vi "SIAM-SIMStack_v3camphase.vi"(7 "Constants":T2={"galvox-Line0"=14800, "GalvoX-Blanking"=15000.0, "galvox-count/pix"=-2.47, "Camera-StartLine"=1, "Camera-Endline"=5000, "Wobbel-total"=4900.0, "SM_ticks"=116, "Trigger_ticks"=100, "galvoxAccel"=10.0, "WobbelAccel"=0.04, "zAccel"=0.05, "z-delay-ticks"=700, "SCMOS-LineSpeed [10µs]"=2.472, "RollingShutter height- Pix"=200} {"SCMOS-LineSpeed [10µs]" format="%#.6f" items=["Fast-285MHz"=0.9175, "Slow-95MHz"=2.7525, "Slow4.2"=2.7766]; "galvox-count/pix" format="%#_5f"}, 8 "error in (no error)":errorcluster, 11 "User":T3={"z-distance_nm"=-200, "#planes"=1, "Digital-out"=enum."Laser1", "NoOfPhaseImages"=7} {"#planes" min=1}) -> (0 "error out":errorcluster, 1 "SIAMScript":T5(array[cluster])=[{"Delay 10µs"=50, "command"=4060086273, "P0"=3, "P1"=1, "P2"=0, "P3"=0, "P4"=0, "P5-ticket"=0}, {"Delay 10µs"=0, "command"=101711937, "P0"=0, "P1"=160563200, "P2"=0, "P3"=0, "P4"=0, "P5-ticket"=0}, {"Delay 10µs"=0, "command"=102760513, "P0"=0, "P1"=985958318, "P2"=0, "P3"=0, "P4"=0, "P5-ticket"=0}, {"Delay 10µs"=0, "command"=3289190402, "P0"=0, "P1"=0, "P2"=0, "P3"=0, "P4"=0, "P5-ticket"=0}, {"Delay 10µs"=1, "command"=4076863488, "P0"=0, "P1"=381040, "P2"=0, "P3"=0, "P4"=0, "P5-ticket"=0}, {"Delay 10µs"=0, "command"=4076863492, "P0"=0, "P1"=0, "P2"=0, "P3"=0, "P4"=0, "P5-ticket"=0}, {"Delay 10µs"=0, "command"=4076863497, "P0"=0, "P1"=1, "P2"=0, "P3"=0, "P4"=0, "P5-ticket"=0}, {"Delay 10µs"=0, "command"=4076863494, "P0"=0, "P1"=0, "P2"=0, "P3"=0, "P4"=0, "P5-ticket"=0}, {"Delay 10µs"=0, "command"=4076863488, "P0"=0, "P1"=40, "P2"=0, "P3"=0, "P4"=0, "P5-ticket"=0}, {"Delay 10µs"=0, "command"=4060086273, "P0"=10, "P1"=-65, "P2"=0, "P3"=0, "P4"=0, "P5-ticket"=0}, {"Delay 10µs"=0, "command"=4076863492, "P0"=10, "P1"=0, "P2"=0, "P3"=0, "P4"=0, "P5-ticket"=0}, {"Delay 10µs"=264, "command"=102760481, "P0"=0, "P1"=0, "P2"=-1047728, "P3"=0, "P4"=0, "P5-ticket"=0}, {"Delay 10µs"=0, "command"=4060086273, "P0"=2, "P1"=7, "P2"=0, "P3"=0, "P4"=0, "P5-ticket"=0}, {"Delay 10µs"=116, "command"=3489660929, "P0"=2097152, "P1"=2097152, "P2"=0, "P3"=0, "P4"=0, "P5-ticket"=0}, {"Delay 10µs"=0, "command"=3489660929, "P0"=1, "P1"=1, "P2"=0, "P3"=0, "P4"=0, "P5-ticket"=0}, {"Delay 10µs"=100, "command"=3489660929, "P0"=1, "P1"=0, "P2"=0, "P3"=0, "P4"=0, "P5-ticket"=0}, {"Delay 10µs"=12638, "command"=3289190402, "P0"=0, "P1"=0, "P2"=0, "P3"=0, "P4"=0, "P5-ticket"=0}, {"Delay 10µs"=1, "command"=4076863488, "P0"=0, "P1"=381040, "P2"=0, "P3"=0, "P4"=0, "P5-ticket"=0}, {"Delay 10µs"=0, "command"=4076863492, "P0"=0, "P1"=0, "P2"=0, "P3"=0, "P4"=0, "P5-ticket"=0}, {"Delay 10µs"=0, "command"=4076863497, "P0"=0, "P1"=1, "P2"=0, "P3"=0, "P4"=0, "P5-ticket"=0}, {"Delay 10µs"=0, "command"=4076863494, "P0"=0, "P1"=0, "P2"=0, "P3"=0, "P4"=0, "P5-ticket"=0}, {"Delay 10µs"=0, "command"=4076863488, "P0"=0, "P1"=40, "P2"=0, "P3"=0, "P4"=0, "P5-ticket"=0}, {"Delay 10µs"=0, "command"=4060086273, "P0"=10, "P1"=-65, "P2"=0, "P3"=0, "P4"=0, "P5-ticket"=0}, {"Delay 10µs"=0, "command"=4076863492, "P0"=10, "P1"=0, "P2"=0, "P3"=0, "P4"=0, "P5-ticket"=0}, {"Delay 10µs"=0, "command"=102760465, "P0"=0, "P1"=794884, "P2"=0, "P3"=0, "P4"=0, "P5-ticket"=0}, {"Delay 10µs"=0, "command"=101711889, "P0"=0, "P1"=42448, "P2"=0, "P3"=0, "P4"=0, "P5-ticket"=0}, {"Delay 10µs"=132, "command"=102760465, "P0"=0, "P1"=-794884, "P2"=0, "P3"=0, "P4"=0, "P5-ticket"=0}, {"Delay 10µs"=0, "command"=101711889, "P0"=0, "P1"=-42448, "P2"=0, "P3"=0, "P4"=0, "P5-ticket"=0}, {"Delay 10µs"=132, "command"=102760465, "P0"=0, "P1"=0, "P2"=0, "P3"=0, "P4"=0, "P5-ticket"=0}, {"Delay 10µs"=0, "command"=101711889, "P0"=0, "P1"=0, "P2"=0, "P3"=0, "P4"=0, "P5-ticket"=0}, {"Delay 10µs"=12855, "command"=3489660929, "P0"=2097152, "P1"=0, "P2"=0, "P3"=0, "P4"=0, "P5-ticket"=0}, {"Delay 10µs"=70, "command"=4043379297, "P0"=-6, "P1"=2, "P2"=1, "P3"=0, "P4"=0, "P5-ticket"=514}, {"Delay 10µs"=50, "command"=104857729, "P0"=-25600, "P1"=0, "P2"=0, "P3"=0, "P4"=0, "P5-ticket"=0}, {"Delay 10µs"=0, "command"=4043379297, "P0"=-43, "P1"=3, "P2"=1, "P3"=0, "P4"=0, "P5-ticket"=515}, {"Delay 10µs"=50, "command"=104857729, "P0"=25600, "P1"=0, "P2"=0, "P3"=0, "P4"=0, "P5-ticket"=0}, {"Delay 10µs"=50, "command"=102760513, "P0"=0, "P1"=983040000, "P2"=0, "P3"=0, "P4"=0, "P5-ticket"=0}, {"Delay 10µs"=10, "command"=4027518991, "P0"=0, "P1"=0, "P2"=0, "P3"=0, "P4"=0, "P5-ticket"=112}] {"command" format="%x" items=["read_x-Motor_status_ticket"=17305600, "init_x-Motor"=17760263, "read_x-Motor_absolute_ticket"=16781312, "move_x-Motor_absolute"=16777217, "move_x-Motor_relative"=16842753, "read_x-Motor_speed"=16977920, "set_x-Motor_speed"=16973825, "read_y-Motor_status_ticket"=18354176, "init_y-Motor"=18808839, "read_y-Motor_absolute_ticket"=17829888, "move_y-Motor_absolute"=17825793, "move_y-Motor_relative"=17891329, "read_y-Motor_speed"=18026496, "set_y-Motor_speed"=18022401, "read_z-Motor_status_ticket"=19402752, "init_z-Motor"=19857415, "stop_z-Motor"=19857423, "start_z-Motor"=19857422, "read_z-Motor_absolute_ticket"=18878464, "move_z-Motor_absolute"=18874369, "move_z-Motor_relative"=18939905, "read_Objective_status_ticket"=20451328, "init_Objective"=20905991, "read_Objective_absolute_ticket"=19927040, "move_Objective_absolute"=19922945, "move_Objective_relative"=19988481, "read_Objective-Motor_speed"=20123648, "set_Objective-Motor_speed"=20119553, "read_Filter_status_ticket"=21499904, "init_Filter"=21954567, "read_Filter_absolute_ticket"=20975616, "move_Filter_absolute"=20971521, "move_Filter_relative"=21037057, "read_Filter-Motor_speed"=21172224, "set_Filter-Motor_speed"=21168129, "read_Trans-Rad_status_ticket"=22548480, "init_Trans-Rad"=23003143, "read_Trans-Rad_absolute_ticket"=22024192, "move_Trans-Rad_absolute"=22020097, "move_Trans-Rad_relative"=22085633, "read_Trans-Motor_speed"=22220800, "set_Trans-Motor_speed"=22216705, "read_FRET_status_ticket"=23597056, "init_FRET"=24051719, "read_FRET_absolute_ticket"=23072768, "move_FRET_absolute"=23068673, "move_FRET_relative"=23134209, "read_FRET-Motor_speed"=23269376, "set_FRET-Motor_speed"=23265281, "read_SI-Rad_status_ticket"=24645632, "init_SI-Rad"=25100295, "read_SI-Rad_absolute_ticket"=24121344, "move_SI-Rad_absolute"=24117249, "move_SI-Rad_relative"=24182785, "read_SI-Rad_speed"=24317952, "set_SI-Rad_speed"=24313857, "I2C-write"=335544337, "I2C-read"=335548433, "UART0-VC-Baud-write"=469958673, "UART0-VC-Baud-read"=469962768, "UART0-VC-write"=469762065, "UART0-VC-write-Var"=469762067, "UART0-VC-read"=469766160, "UART0-VC-read-Var"=469766162, "UART1-TSM-Baud-read"=486739984, "UART1-TSM-write"=486539281, "UART1-TSM-write-ticket"=486543377, "UART1-TSM-write-var-binary"=486539283, "UART1-TSM-write-var-binary-ticket"=486543379, "UART1-TSM-read"=486543376, "UART1-TSM-read-var-binary"=486543378, "UART2-write"=503316497, "UART2-read"=503320592, "USB-UART0-write"=536870929, "USB-UART0-read"=536875024, "USB-UART0-Float-Bitschift"=537133073, "USB-UART0-read-Float"=536875234, "USB-UART0-write-Float"=536871139, "USB-UART0-read-Float"=536875250, "USB-UART0-write-Float"=536871155, "end_no_ticket"=4027514895, "end_ticket"=4027518991, "IO-read_bank0"=3489665024, "IO-write_bank0"=3489660929, "IO-read_bank1"=3506442240, "IO-write_bank1"=3506438145, "DA0-0_LED365"=2684354561, "DA0-1_LED385"=2685403137, "DA0-2_LED440"=2686451713, "DA0-3_LED470"=2687500289, "DA0-4_LED510"=2688548865, "DA0-5_LED550"=2689597441, "DA0-6_LED590"=2690646017, "DA0-7_LED640"=2691694593, "DA1-0_LED-R"=2701131777, "DA1-1_LED-G"=2702180353, "DA1-2_LED-B"=2703228929, "DA1-3_LED-AF"=2704277505, "DA1-4"=2705326081, "DA1-5"=2706374657, "DA1-6"=2707423233, "DA1-7"=2708471809, "DA2-Laser0"=2717908993, "DA2-Laser1"=2718957569, "DA2-Laser2"=2720006145, "DA2-Laser3"=2721054721, "DA2-Laser4"=2722103297, "Analog-read_AD0-0"=2818576384, "Analog-read-store_AD0-0"=2818572290, "IO-delay_bank0"=3489923073, "IO-delay_bank0_fromVar"=3489923075, "read_cam_clock"=3289124864, "store_cam_clock"=3289120770, "read_cam_phase"=3289190400, "store_cam_phase"=3289186306, "store_cam_phase-t"=3289190402, "Read ticks"=4027518976, "Read ticks to var"=4027518978, "Read IP"=4043313152, "Read IP into var"=4043313154, "Set IP from var"=4043309059, "Set IP from var, relative"=4043313155, "decrement_branchRel_if_equal"=4043374945, "decrement_branchRel_if_greaterequal"=4043375201, "decrement_branchRel_if_greaterequal_withTicket"=4043379297, "decrement_branchRel_if_smaller"=4043375457, "increment_branchRel_if_smaller"=4043375473, "readVar"=4060090368, "writeVar"=4060086273, "copyVar0_from_var1"=4060086275, "math_addToVariable"=4076863488, "math_addVToVariable"=4076863489, "math_subToVariable"=4076863490, "math_subVToVariable"=4076863491, "math_multToVariable"=4076863492, "math_multvToVariable"=4076863493, "math_divideToVariable"=4076863494, "math_divideVToVariable"=4076863495, "math_modToVariable"=4076863496, "math_modVToVariable"=4076863497, "logic_and"=4093640704, "logic_or"=4093640706, "logic_xor"=4093640708, "bitshift"=4093640712, "set_1Galvo"=101712113, "set_x-Galvo"=102760689, "set_y-Galvo"=103809265, "set_z-Fokus"=104857841, "set_1Galvo_position-only"=101711937, "set_x-Galvo_position-only"=102760513, "set_y-Galvo_position-only"=103809089, "set_z-Fokus_position-only"=104857665, "set_x-Galvo_position-only_ticket"=102764609, "set_y-Galvo_position-only_ticket"=103813185, "set_z-Fokus_position-only_ticket"=104861761, "set_1Galvo_relativ-only"=101712001, "set_x-Galvo_relativ-only"=102760577, "set_y-Galvo_relativ-only"=103809153, "set_z-Fokus_relativ-only"=104857729, "set_1Galvo_speed-only"=101711905, "set_x-Galvo_speed-only"=102760481, "set_y-Galvo_speed-only"=103809057, "set_z-Fokus_speed-only"=104857633, "set_1Galvo_acc-only"=101711889, "set_x-Galvo_acc-only"=102760465, "set_y-Galvo_acc-only"=103809041, "set_z-Fokus_acc-only"=104857617, "read_1Galvo_ticket"=101716032, "read_x-Galvo_ticket"=102764608, "read_y-Galvo_ticket"=103813184, "read_z-Focus_ticket"=104861760, "x-Galvo_pos_fromVar"=102760515, "y-Galvo_pos_fromVar"=103809091, "z-Focus_pos_fromVar"=104857667, "Servo0"=67108865, "Servo0-enable"=68091911, "Servo0-disable"=68091919, "Servo1"=68157441, "Servo1-enable"=69140487, "Servo1-disable"=69140495, "Servo2-enable"=70189063, "Servo2"=69206017, "Servo3-enable"=71237639, "Servo3"=70254593, "xEncoder-Enable"=202309639, "xEncoder-Bits"=201523201, "xEncoder-Read"=201330688, "xEncoder-Read"=201326594, "xEncoder-Read-ticket"=201330690, "yEncoder-Enable"=203358215, "yEncoder-Bits"=202571777, "yEncoder-Read"=202379264, "yEncoder-Read"=202375170, "yEncoder-Read-ticket"=202379266]}, 2 "Camera":T1={"Camera-Exposure"=0.0, "CameraImages"=7})   [LabVIEW 2011]
uses:
  SIAM_command.ctl
panel:
  out "phase a":dbl=0.04048114735137636
  out "galvo a":dbl=0.7580607172293603
  out "GalvoMove":dbl=-12844.599514563108
  out "PredictionTime":u32=381
  out "FrameClock":u32=13119
  out "CamTics":u32=12855
  out "x vel":dbl=-0.9991909385113269
  out "~x-move":dbl=12841.530000000002
  out "xgalvoend":dbl=2202.999999999998
  out "xgalvostart":dbl=15044.53
  out "expected xduration":dbl=71.67016115511393
  out "expected  Wduration":dbl=264.5751311064591
  out "size(s)":i32=37
  out "WobShift":dbl=700.0
  out "Half Turn_ticks":u32=132
  # "todo:\ntest! nö klinkt 12........34 \nversion ohne phase?\nversion mit galvo1 parallel galvox!"
  # "var0=phase\nvar1=clock256\nvar 2 =linecounter \nvar 3 =framecounter"
  # "<-- user inputs --------------------------- constants ---->"
  # "Pixel definition: 0\nmiddel: lines\nbottom +2lines"
  # "alles umstellen auf count und Pixel und 10µs !!!"
  # "wobbler shift(7)=SQRT(7)*pitch"
  # "lineclock read slow=AD99E =711070 =/256=27.77617"
  # "a gerechnet wobbler~3.7, x~98, eher /2\nz~6ms/2µm"
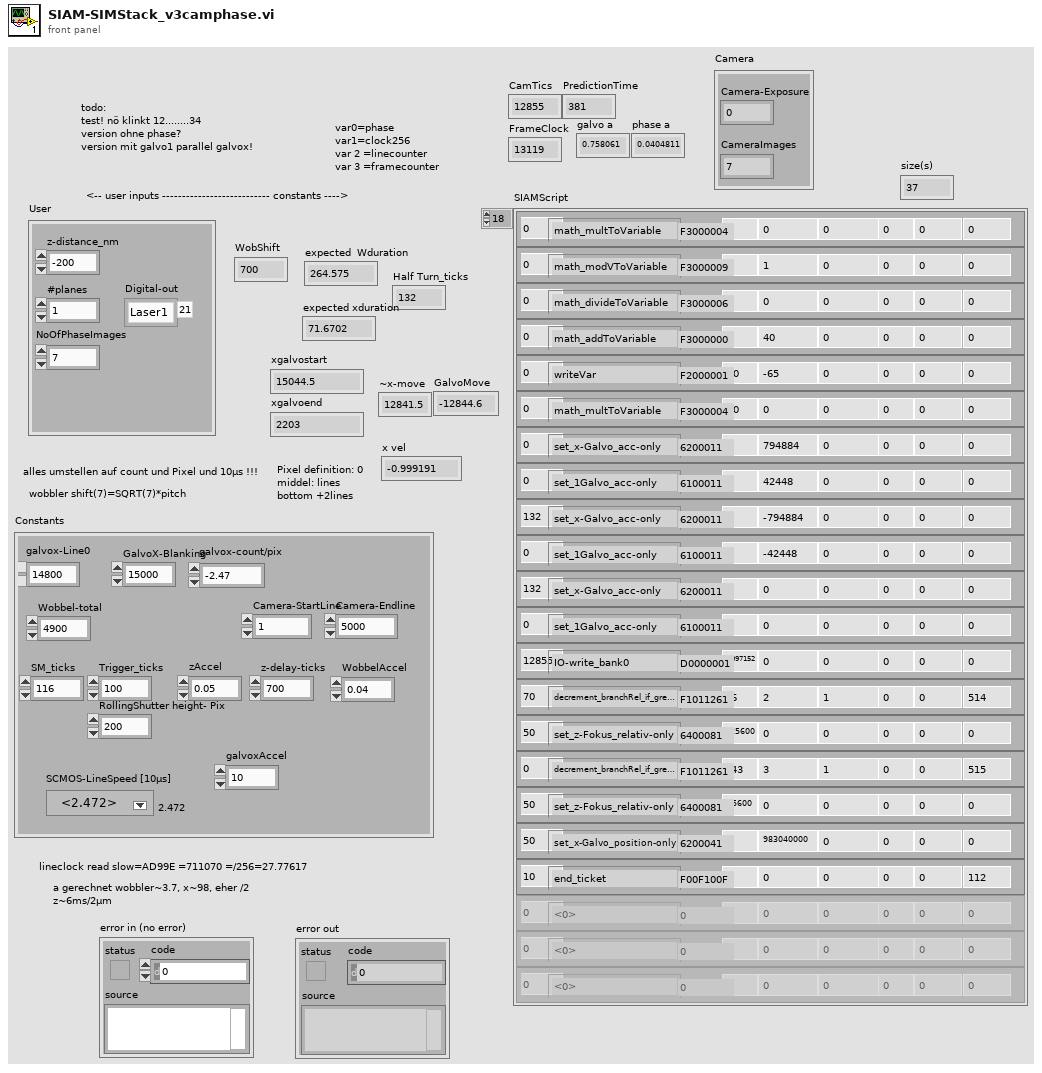
[diagram p1: front panel]
types:
  T1 = cluster{"Camera-Exposure":dbl, "CameraImages":u16}
  T2 = cluster{"galvox-Line0":i16, "GalvoX-Blanking":dbl, "galvox-count/pix":dbl, "Camera-StartLine":u32, "Camera-Endline":u32, "Wobbel-total":dbl, "SM_ticks":u32, "Trigger_ticks":u32, "galvoxAccel":dbl, "WobbelAccel":dbl, "zAccel":dbl, "z-delay-ticks":u32, "SCMOS-LineSpeed [10µs]":dbl, "RollingShutter height- Pix":u16}
  T3 = cluster{"z-distance_nm":i32, "#planes":u16, "Digital-out":enum8{"cam1", "cam1-ready?", "cam2", "cam2-ready?", "tmsx?", "tsmy?", "tsm3?", "lid?", "led1", "led2", "led3", "led4", "led5", "led6", "led7", "led8", "durchR", "durchG", "durchB", "AF", "Laser0", "Laser1", "Laser2", "Laser3", "Laser4", "LaserX", "TrigOut", "SMB1", ""}, "NoOfPhaseImages":u16}
  T4 = typedef "SIAM_command.ctl" = u32
  T5 = cluster{"Delay 10µs":u32, "command":T4, "P0":i32, "P1":i32, "P2":i32, "P3":i32, "P4":i32, "P5-ticket":i32}[]
  T6 = enum8{"Ch0", "Ch1", "x-Galvo", "y-Galvo", "z-Focus"}
  T7 = cluster{"Delay 10µs":u32, "command":T4, "P0":i32, "P1":i32, "P2":i32, "P3":i32, "P4":i32, "P5-ticket":i32}
  T8 = enum8{"cam1", "cam1-ready?", "cam2", "cam2-ready?", "tmsx?", "tsmy?", "tsm3?", "lid?", "led1", "led2", "led3", "led4", "led5", "led6", "led7", "led8", "durchR", "durchG", "durchB", "AF", "Laser0", "Laser1", "Laser2", "Laser3", "Laser4", "LaserX", "TrigOut", "SMB1", ""}
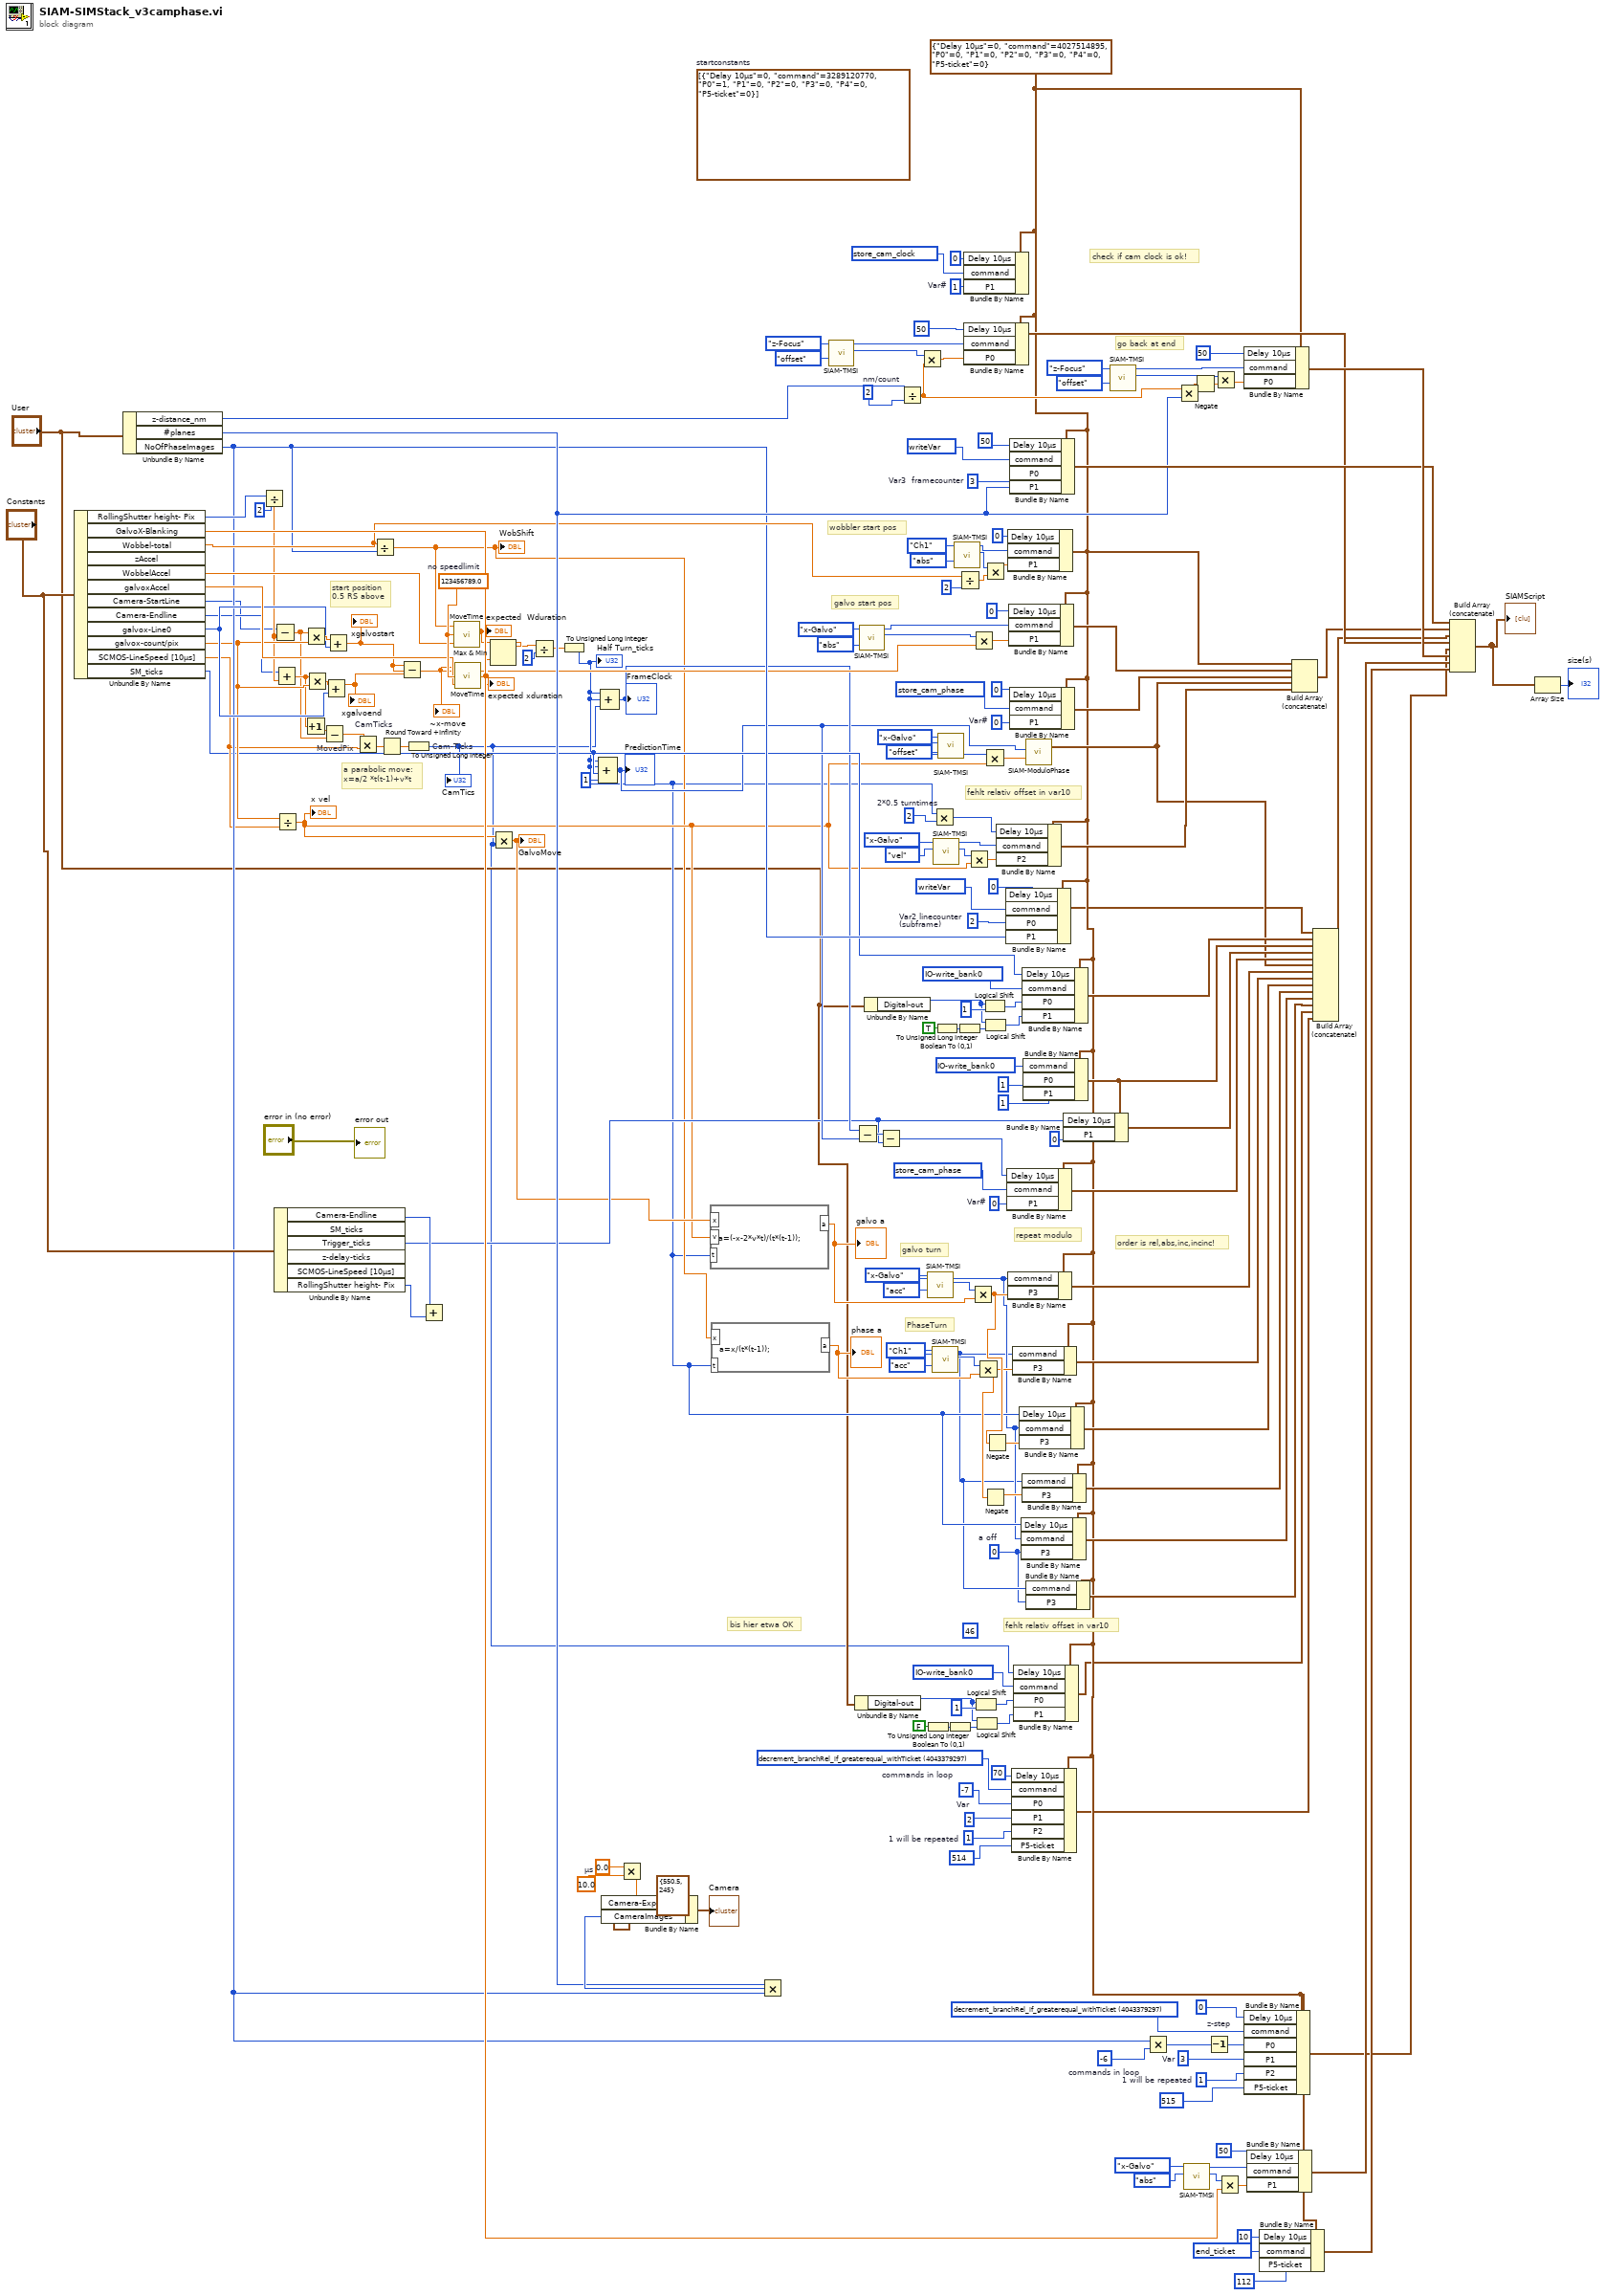
[diagram p0: block diagram]
diagram:
  (unwired) u32 46 ("Delay 10µs")
  w14 = T4 3489660929 items=["read_x-Motor_status_ticket"=17305600, "init_x-Motor"=17760263, "read_x-Motor_absolute_ticket"=16781312, "move_x-Motor_absolute"=16777217, "move_x-Motor_relative"=16842753, "read_y-Motor_status_ticket"=18354176, "init_y-Motor"=18808839, "read_y-Motor_absolute_ticket"=17829888, "move_y-Motor_absolute"=17825793, "move_y-Motor_relative"=17891329, "read_z-Motor_status_ticket"=19402752, "init_z-Motor"=19857415, "stop_z-Motor"=19857423, "start_z-Motor"=19857422, "read_z-Motor_absolute_ticket"=18878464, "move_z-Motor_absolute"=18874369, "move_z-Motor_relative"=18939905, "end_no_ticket"=4027514895, "end_ticket"=4027518991, "IO-read_bank0"=3489665024, "IO-write_bank0"=3489660929, "IO-read_bank1"=3506442240, "IO-write_bank1"=3506438145, "IO-delay_bank0"=3489923073, "IO-delay_bank0_fromVar"=3489923075, "read_cam_clock"=3289124864, "store_cam_clock"=3289120770, "read_cam_phase"=3289190400, "set_cam_deadtime"=3288989697, "set_cam_10uscycles"=3289055233, "set_cam_10uscycles_fromVariable"=3289055235, "calc_cam"=3289317386, "store_cam_Var"=3289251842, "math_addToVariable"=4060086278, "readVar"=4060090368, "writeVar"=4060086273, "copyVar"=4060086276, "decrement_branchRel_if_equal"=4043374945, "decrement_branchRel_if_greaterequal"=4043375201, "decrement_branchRel_if_greaterequal_withTicket"=4043379297, "decrement_branchRel_if_smaller"=4043375457, "increment_branchRel_if_smaller"=4043375473, "set_x-Galvo"=1612710129, "set_y-Galvo"=1613758705, "set_z-Fokus"=1614807281, "set_x-Galvo_position-only"=1612709953, "set_y-Galvo_position-only"=1613758529, "set_z-Fokus_position-only"=1614807105, "set_x-Galvo_position-only_ticket"=1612714049, "set_y-Galvo_position-only_ticket"=1613762625, "set_z-Fokus_position-only_ticket"=1614811201, "read_x-Galvo_ticket"=1612714048, "read_y-Galvo_ticket"=1613762624, "read_z-Focus_ticket"=1614811200, "x-Galvo_pos_fromVar"=1612709955, "y-Galvo_pos_fromVar"=1613758531, "z-Focus_pos_fromVar"=1614807107] ("command")
  w18 = 0  # a off
  w52 = 0  # Var#
  w53 = T4 3289190402 items=["read_x-Motor_status_ticket"=17305600, "init_x-Motor"=17760263, "read_x-Motor_absolute_ticket"=16781312, "move_x-Motor_absolute"=16777217, "move_x-Motor_relative"=16842753, "read_x-Motor_speed"=16977920, "set_x-Motor_speed"=16973825, "read_y-Motor_status_ticket"=18354176, "init_y-Motor"=18808839, "read_y-Motor_absolute_ticket"=17829888, "move_y-Motor_absolute"=17825793, "move_y-Motor_relative"=17891329, "read_y-Motor_speed"=18026496, "set_y-Motor_speed"=18022401, "read_z-Motor_status_ticket"=19402752, "init_z-Motor"=19857415, "stop_z-Motor"=19857423, "start_z-Motor"=19857422, "read_z-Motor_absolute_ticket"=18878464, "move_z-Motor_absolute"=18874369, "move_z-Motor_relative"=18939905, "read_Objective_status_ticket"=20451328, "init_Objective"=20905991, "read_Objective_absolute_ticket"=19927040, "move_Objective_absolute"=19922945, "move_Objective_relative"=19988481, "read_Objective-Motor_speed"=20123648, "set_Objective-Motor_speed"=20119553, "read_Filter_status_ticket"=21499904, "init_Filter"=21954567, "read_Filter_absolute_ticket"=20975616, "move_Filter_absolute"=20971521, "move_Filter_relative"=21037057, "read_Filter-Motor_speed"=21172224, "set_Filter-Motor_speed"=21168129, "read_Trans-Rad_status_ticket"=22548480, "init_Trans-Rad"=23003143, "read_Trans-Rad_absolute_ticket"=22024192, "move_Trans-Rad_absolute"=22020097, "move_Trans-Rad_relative"=22085633, "read_Trans-Motor_speed"=22220800, "set_Trans-Motor_speed"=22216705, "read_FRET_status_ticket"=23597056, "init_FRET"=24051719, "read_FRET_absolute_ticket"=23072768, "move_FRET_absolute"=23068673, "move_FRET_relative"=23134209, "read_FRET-Motor_speed"=23269376, "set_FRET-Motor_speed"=23265281, "read_SI-Rad_status_ticket"=24645632, "init_SI-Rad"=25100295, "read_SI-Rad_absolute_ticket"=24121344, "move_SI-Rad_absolute"=24117249, "move_SI-Rad_relative"=24182785, "read_SI-Rad_speed"=24317952, "set_SI-Rad_speed"=24313857, "I2C-write"=335544321, "I2C-read"=335548416, "end_no_ticket"=4027514895, "end_ticket"=4027518991, "IO-read_bank0"=3489665024, "IO-write_bank0"=3489660929, "IO-read_bank1"=3506442240, "IO-write_bank1"=3506438145, "DA0-0_LED365"=2684354561, "DA0-1_LED385"=2685403137, "DA0-2_LED440"=2686451713, "DA0-3_LED470"=2687500289, "DA0-4_LED510"=2688548865, "DA0-5_LED550"=2689597441, "DA0-6_LED590"=2690646017, "DA0-7_LED640"=2691694593, "DA1-0_LED-R"=2701131777, "DA1-1_LED-G"=2702180353, "DA1-2_LED-B"=2703228929, "DA1-3_LED-AF"=2704277505, "DA1-4"=2705326081, "DA1-5"=2706374657, "DA1-6"=2707423233, "DA1-7"=2708471809, "DA2-Laser0"=2717908993, "DA2-Laser1"=2718957569, "DA2-Laser2"=2720006145, "DA2-Laser3"=2721054721, "DA2-Laser4"=2722103297, "Analog-read_AD0-0"=2818576384, "Analog-read-store_AD0-0"=2818572290, "IO-delay_bank0"=3489923073, "IO-delay_bank0_fromVar"=3489923075, "read_cam_clock"=3289124864, "store_cam_clock"=3289120770, "read_cam_phase"=3289190400, "store_cam_phase"=3289190402, "Read ticks"=4027518976, "Read ticks to var"=4027518978, "Read IP"=4043313152, "Read IP into var"=4043313154, "Set IP from var"=4043309059, "Set IP from var, relative"=4043313155, "decrement_branchRel_if_equal"=4043374945, "decrement_branchRel_if_greaterequal"=4043375201, "decrement_branchRel_if_greaterequal_withTicket"=4043379297, "decrement_branchRel_if_smaller"=4043375457, "increment_branchRel_if_smaller"=4043375473, "readVar"=4060090368, "writeVar"=4060086273, "readVar_and_copy_to_var2"=4060086275, "loadVar2_andcopy_var1"=4060086276, "math_addToVariable"=4076863488, "math_addVToVariable"=4076863489, "math_subToVariable"=4076863490, "math_subVToVariable"=4076863491, "math_multToVariable"=4076863492, "math_multvToVariable"=4076863493, "math_divideToVariable"=4076863494, "math_divideVToVariable"=4076863495, "math_modToVariable"=4076863496, "math_modVToVariable"=4076863497, "logic_and"=4093640704, "logic_or"=4093640706, "logic_xor"=4093640708, "set_1Galvo"=101712113, "set_x-Galvo"=102760689, "set_y-Galvo"=103809265, "set_z-Fokus"=104857841, "set_1Galvo_position-only"=101711937, "set_x-Galvo_position-only"=102760513, "set_y-Galvo_position-only"=103809089, "set_z-Fokus_position-only"=104857665, "set_x-Galvo_position-only_ticket"=102764609, "set_y-Galvo_position-only_ticket"=103813185, "set_z-Fokus_position-only_ticket"=104861761, "set_x-Galvo_relativ-only"=102760577, "set_y-Galvo_relativ-only"=103809153, "set_z-Fokus_relativ-only"=104857729, "set_x-Galvo_speed-only"=102760481, "set_y-Galvo_speed-only"=103809057, "set_z-Fokus_speed-only"=104857633, "read_1Galvo_ticket"=101716032, "read_x-Galvo_ticket"=102764608, "read_y-Galvo_ticket"=103813184, "read_z-Focus_ticket"=104861760, "x-Galvo_pos_fromVar"=102760515, "y-Galvo_pos_fromVar"=103809091, "z-Focus_pos_fromVar"=104857667, "Servo0"=67108865, "Servo0-enable"=68091911, "Servo0-disable"=68091919, "Servo1"=68157441, "Servo1-enable"=69140487, "Servo1-disable"=69140495, "EnablePower0-SM"=2148466695, "DisablePower0-SM"=2148466703, "EnablePower1-Thermo1"=2149515271, "DisablePower1-Thermo1"=2149515279, "EnablePower2-Cam"=2150563847, "DisablePower2-Cam"=2150563855, "EnablePower3-Thermo2"=2151612423, "DisablePower3-Thermo2"=2151612431, "EnablePower4-Laser0"=2152660999, "DisablePower4-Laser0"=2152661007, "EnablePower5"=2153709575, "DisablePower5"=2153709583, "EnablePower6-Laser1"=2154758151, "DisablePower6-Laser1"=2154758159, "EnablePower7-SAM"=2155806727, "DisablePower7-SAM"=2155806735, "EnablePower8-Laser2"=2156855303, "DisablePower8-Laser2"=2156855311, "EnablePower9-TSM"=2157903879, "DisablePower9-TSM"=2157903887, "EnablePower10-Laser3"=2158952455, "DisablePower10-Laser3"=2158952463, "EnablePower11-Servo"=2160001031, "DisablePower11-Servo"=2160001039, "EnablePower12-Laser4"=2161049607, "DisablePower12-Laser4"=2161049615, "EnableSMPower2-DCC22"=2167341063, "DisableSMPower2-DCC22"=2167341071, "EnableSMPower3-6220"=2168389639, "DisableSMPower3-6220"=2168389647, "EnableSMPower4-6210"=2169438215, "DisableSMPower4-6210"=2169438223] ("command")
  w62 = T4 3489660929 items=["read_x-Motor_status_ticket"=17305600, "init_x-Motor"=17760263, "read_x-Motor_absolute_ticket"=16781312, "move_x-Motor_absolute"=16777217, "move_x-Motor_relative"=16842753, "read_y-Motor_status_ticket"=18354176, "init_y-Motor"=18808839, "read_y-Motor_absolute_ticket"=17829888, "move_y-Motor_absolute"=17825793, "move_y-Motor_relative"=17891329, "read_z-Motor_status_ticket"=19402752, "init_z-Motor"=19857415, "stop_z-Motor"=19857423, "start_z-Motor"=19857422, "read_z-Motor_absolute_ticket"=18878464, "move_z-Motor_absolute"=18874369, "move_z-Motor_relative"=18939905, "end_no_ticket"=4027514895, "end_ticket"=4027518991, "IO-read_bank0"=3489665024, "IO-write_bank0"=3489660929, "IO-read_bank1"=3506442240, "IO-write_bank1"=3506438145, "IO-delay_bank0"=3489923073, "IO-delay_bank0_fromVar"=3489923075, "read_cam_clock"=3289124864, "store_cam_clock"=3289120770, "read_cam_phase"=3289190400, "set_cam_deadtime"=3288989697, "set_cam_10uscycles"=3289055233, "set_cam_10uscycles_fromVariable"=3289055235, "calc_cam"=3289317386, "store_cam_Var"=3289251842, "math_addToVariable"=4060086278, "readVar"=4060090368, "writeVar"=4060086273, "copyVar"=4060086276, "decrement_branchRel_if_equal"=4043374945, "decrement_branchRel_if_greaterequal"=4043375201, "decrement_branchRel_if_greaterequal_withTicket"=4043379297, "decrement_branchRel_if_smaller"=4043375457, "increment_branchRel_if_smaller"=4043375473, "set_x-Galvo"=1612710129, "set_y-Galvo"=1613758705, "set_z-Fokus"=1614807281, "set_x-Galvo_position-only"=1612709953, "set_y-Galvo_position-only"=1613758529, "set_z-Fokus_position-only"=1614807105, "set_x-Galvo_position-only_ticket"=1612714049, "set_y-Galvo_position-only_ticket"=1613762625, "set_z-Fokus_position-only_ticket"=1614811201, "read_x-Galvo_ticket"=1612714048, "read_y-Galvo_ticket"=1613762624, "read_z-Focus_ticket"=1614811200, "x-Galvo_pos_fromVar"=1612709955, "y-Galvo_pos_fromVar"=1613758531, "z-Focus_pos_fromVar"=1614807107] ("command")
  w6 = T7 {"Delay 10µs"=0, "command"=4027514895, "P0"=0, "P1"=0, "P2"=0, "P3"=0, "P4"=0, "P5-ticket"=0} ("Cluster")
  (unwired) T5 [{"Delay 10µs"=0, "command"=3289120770, "P0"=1, "P1"=0, "P2"=0, "P3"=0, "P4"=0, "P5-ticket"=0}]  # startconstants
  w87 = 1  # Var#
  w88 = T4 3289120770 items=["read_x-Motor_status_ticket"=17305600, "init_x-Motor"=17760263, "read_x-Motor_absolute_ticket"=16781312, "move_x-Motor_absolute"=16777217, "move_x-Motor_relative"=16842753, "read_x-Motor_speed"=16977920, "set_x-Motor_speed"=16973825, "read_y-Motor_status_ticket"=18354176, "init_y-Motor"=18808839, "read_y-Motor_absolute_ticket"=17829888, "move_y-Motor_absolute"=17825793, "move_y-Motor_relative"=17891329, "read_y-Motor_speed"=18026496, "set_y-Motor_speed"=18022401, "read_z-Motor_status_ticket"=19402752, "init_z-Motor"=19857415, "stop_z-Motor"=19857423, "start_z-Motor"=19857422, "read_z-Motor_absolute_ticket"=18878464, "move_z-Motor_absolute"=18874369, "move_z-Motor_relative"=18939905, "read_Objective_status_ticket"=20451328, "init_Objective"=20905991, "read_Objective_absolute_ticket"=19927040, "move_Objective_absolute"=19922945, "move_Objective_relative"=19988481, "read_Objective-Motor_speed"=20123648, "set_Objective-Motor_speed"=20119553, "read_Filter_status_ticket"=21499904, "init_Filter"=21954567, "read_Filter_absolute_ticket"=20975616, "move_Filter_absolute"=20971521, "move_Filter_relative"=21037057, "read_Filter-Motor_speed"=21172224, "set_Filter-Motor_speed"=21168129, "read_Trans-Rad_status_ticket"=22548480, "init_Trans-Rad"=23003143, "read_Trans-Rad_absolute_ticket"=22024192, "move_Trans-Rad_absolute"=22020097, "move_Trans-Rad_relative"=22085633, "read_Trans-Motor_speed"=22220800, "set_Trans-Motor_speed"=22216705, "read_FRET_status_ticket"=23597056, "init_FRET"=24051719, "read_FRET_absolute_ticket"=23072768, "move_FRET_absolute"=23068673, "move_FRET_relative"=23134209, "read_FRET-Motor_speed"=23269376, "set_FRET-Motor_speed"=23265281, "read_SI-Rad_status_ticket"=24645632, "init_SI-Rad"=25100295, "read_SI-Rad_absolute_ticket"=24121344, "move_SI-Rad_absolute"=24117249, "move_SI-Rad_relative"=24182785, "read_SI-Rad_speed"=24317952, "set_SI-Rad_speed"=24313857, "I2C-write"=335544321, "I2C-read"=335548416, "end_no_ticket"=4027514895, "end_ticket"=4027518991, "IO-read_bank0"=3489665024, "IO-write_bank0"=3489660929, "IO-read_bank1"=3506442240, "IO-write_bank1"=3506438145, "DA0-0_LED365"=2684354561, "DA0-1_LED385"=2685403137, "DA0-2_LED440"=2686451713, "DA0-3_LED470"=2687500289, "DA0-4_LED510"=2688548865, "DA0-5_LED550"=2689597441, "DA0-6_LED590"=2690646017, "DA0-7_LED640"=2691694593, "DA1-0_LED-R"=2701131777, "DA1-1_LED-G"=2702180353, "DA1-2_LED-B"=2703228929, "DA1-3_LED-AF"=2704277505, "DA1-4"=2705326081, "DA1-5"=2706374657, "DA1-6"=2707423233, "DA1-7"=2708471809, "DA2-Laser0"=2717908993, "DA2-Laser1"=2718957569, "DA2-Laser2"=2720006145, "DA2-Laser3"=2721054721, "DA2-Laser4"=2722103297, "Analog-read_AD0-0"=2818576384, "Analog-read-store_AD0-0"=2818572290, "IO-delay_bank0"=3489923073, "IO-delay_bank0_fromVar"=3489923075, "read_cam_clock"=3289124864, "store_cam_clock"=3289120770, "read_cam_phase"=3289190400, "store_cam_phase"=3289190402, "Read ticks"=4027518976, "Read ticks to var"=4027518978, "Read IP"=4043313152, "Read IP into var"=4043313154, "Set IP from var"=4043309059, "Set IP from var, relative"=4043313155, "decrement_branchRel_if_equal"=4043374945, "decrement_branchRel_if_greaterequal"=4043375201, "decrement_branchRel_if_greaterequal_withTicket"=4043379297, "decrement_branchRel_if_smaller"=4043375457, "increment_branchRel_if_smaller"=4043375473, "readVar"=4060090368, "writeVar"=4060086273, "readVar_and_copy_to_var2"=4060086275, "loadVar2_andcopy_var1"=4060086276, "math_addToVariable"=4076863488, "math_addVToVariable"=4076863489, "math_subToVariable"=4076863490, "math_subVToVariable"=4076863491, "math_multToVariable"=4076863492, "math_multvToVariable"=4076863493, "math_divideToVariable"=4076863494, "math_divideVToVariable"=4076863495, "math_modToVariable"=4076863496, "math_modVToVariable"=4076863497, "logic_and"=4093640704, "logic_or"=4093640706, "logic_xor"=4093640708, "set_1Galvo"=101712113, "set_x-Galvo"=102760689, "set_y-Galvo"=103809265, "set_z-Fokus"=104857841, "set_1Galvo_position-only"=101711937, "set_x-Galvo_position-only"=102760513, "set_y-Galvo_position-only"=103809089, "set_z-Fokus_position-only"=104857665, "set_x-Galvo_position-only_ticket"=102764609, "set_y-Galvo_position-only_ticket"=103813185, "set_z-Fokus_position-only_ticket"=104861761, "set_x-Galvo_relativ-only"=102760577, "set_y-Galvo_relativ-only"=103809153, "set_z-Fokus_relativ-only"=104857729, "set_x-Galvo_speed-only"=102760481, "set_y-Galvo_speed-only"=103809057, "set_z-Fokus_speed-only"=104857633, "read_1Galvo_ticket"=101716032, "read_x-Galvo_ticket"=102764608, "read_y-Galvo_ticket"=103813184, "read_z-Focus_ticket"=104861760, "x-Galvo_pos_fromVar"=102760515, "y-Galvo_pos_fromVar"=103809091, "z-Focus_pos_fromVar"=104857667, "Servo0"=67108865, "Servo0-enable"=68091911, "Servo0-disable"=68091919, "Servo1"=68157441, "Servo1-enable"=69140487, "Servo1-disable"=69140495, "EnablePower0-SM"=2148466695, "DisablePower0-SM"=2148466703, "EnablePower1-Thermo1"=2149515271, "DisablePower1-Thermo1"=2149515279, "EnablePower2-Cam"=2150563847, "DisablePower2-Cam"=2150563855, "EnablePower3-Thermo2"=2151612423, "DisablePower3-Thermo2"=2151612431, "EnablePower4-Laser0"=2152660999, "DisablePower4-Laser0"=2152661007, "EnablePower5"=2153709575, "DisablePower5"=2153709583, "EnablePower6-Laser1"=2154758151, "DisablePower6-Laser1"=2154758159, "EnablePower7-SAM"=2155806727, "DisablePower7-SAM"=2155806735, "EnablePower8-Laser2"=2156855303, "DisablePower8-Laser2"=2156855311, "EnablePower9-TSM"=2157903879, "DisablePower9-TSM"=2157903887, "EnablePower10-Laser3"=2158952455, "DisablePower10-Laser3"=2158952463, "EnablePower11-Servo"=2160001031, "DisablePower11-Servo"=2160001039, "EnablePower12-Laser4"=2161049607, "DisablePower12-Laser4"=2161049615, "EnableSMPower2-DCC22"=2167341063, "DisableSMPower2-DCC22"=2167341071, "EnableSMPower3-6220"=2168389639, "DisableSMPower3-6220"=2168389647, "EnableSMPower4-6210"=2169438215, "DisableSMPower4-6210"=2169438223] ("command")
  w91 = 0  # Var#
  w92 = T4 3289190402 items=["read_x-Motor_status_ticket"=17305600, "init_x-Motor"=17760263, "read_x-Motor_absolute_ticket"=16781312, "move_x-Motor_absolute"=16777217, "move_x-Motor_relative"=16842753, "read_x-Motor_speed"=16977920, "set_x-Motor_speed"=16973825, "read_y-Motor_status_ticket"=18354176, "init_y-Motor"=18808839, "read_y-Motor_absolute_ticket"=17829888, "move_y-Motor_absolute"=17825793, "move_y-Motor_relative"=17891329, "read_y-Motor_speed"=18026496, "set_y-Motor_speed"=18022401, "read_z-Motor_status_ticket"=19402752, "init_z-Motor"=19857415, "stop_z-Motor"=19857423, "start_z-Motor"=19857422, "read_z-Motor_absolute_ticket"=18878464, "move_z-Motor_absolute"=18874369, "move_z-Motor_relative"=18939905, "read_Objective_status_ticket"=20451328, "init_Objective"=20905991, "read_Objective_absolute_ticket"=19927040, "move_Objective_absolute"=19922945, "move_Objective_relative"=19988481, "read_Objective-Motor_speed"=20123648, "set_Objective-Motor_speed"=20119553, "read_Filter_status_ticket"=21499904, "init_Filter"=21954567, "read_Filter_absolute_ticket"=20975616, "move_Filter_absolute"=20971521, "move_Filter_relative"=21037057, "read_Filter-Motor_speed"=21172224, "set_Filter-Motor_speed"=21168129, "read_Trans-Rad_status_ticket"=22548480, "init_Trans-Rad"=23003143, "read_Trans-Rad_absolute_ticket"=22024192, "move_Trans-Rad_absolute"=22020097, "move_Trans-Rad_relative"=22085633, "read_Trans-Motor_speed"=22220800, "set_Trans-Motor_speed"=22216705, "read_FRET_status_ticket"=23597056, "init_FRET"=24051719, "read_FRET_absolute_ticket"=23072768, "move_FRET_absolute"=23068673, "move_FRET_relative"=23134209, "read_FRET-Motor_speed"=23269376, "set_FRET-Motor_speed"=23265281, "read_SI-Rad_status_ticket"=24645632, "init_SI-Rad"=25100295, "read_SI-Rad_absolute_ticket"=24121344, "move_SI-Rad_absolute"=24117249, "move_SI-Rad_relative"=24182785, "read_SI-Rad_speed"=24317952, "set_SI-Rad_speed"=24313857, "I2C-write"=335544321, "I2C-read"=335548416, "end_no_ticket"=4027514895, "end_ticket"=4027518991, "IO-read_bank0"=3489665024, "IO-write_bank0"=3489660929, "IO-read_bank1"=3506442240, "IO-write_bank1"=3506438145, "DA0-0_LED365"=2684354561, "DA0-1_LED385"=2685403137, "DA0-2_LED440"=2686451713, "DA0-3_LED470"=2687500289, "DA0-4_LED510"=2688548865, "DA0-5_LED550"=2689597441, "DA0-6_LED590"=2690646017, "DA0-7_LED640"=2691694593, "DA1-0_LED-R"=2701131777, "DA1-1_LED-G"=2702180353, "DA1-2_LED-B"=2703228929, "DA1-3_LED-AF"=2704277505, "DA1-4"=2705326081, "DA1-5"=2706374657, "DA1-6"=2707423233, "DA1-7"=2708471809, "DA2-Laser0"=2717908993, "DA2-Laser1"=2718957569, "DA2-Laser2"=2720006145, "DA2-Laser3"=2721054721, "DA2-Laser4"=2722103297, "Analog-read_AD0-0"=2818576384, "Analog-read-store_AD0-0"=2818572290, "IO-delay_bank0"=3489923073, "IO-delay_bank0_fromVar"=3489923075, "read_cam_clock"=3289124864, "store_cam_clock"=3289120770, "read_cam_phase"=3289190400, "store_cam_phase"=3289190402, "Read ticks"=4027518976, "Read ticks to var"=4027518978, "Read IP"=4043313152, "Read IP into var"=4043313154, "Set IP from var"=4043309059, "Set IP from var, relative"=4043313155, "decrement_branchRel_if_equal"=4043374945, "decrement_branchRel_if_greaterequal"=4043375201, "decrement_branchRel_if_greaterequal_withTicket"=4043379297, "decrement_branchRel_if_smaller"=4043375457, "increment_branchRel_if_smaller"=4043375473, "readVar"=4060090368, "writeVar"=4060086273, "readVar_and_copy_to_var2"=4060086275, "loadVar2_andcopy_var1"=4060086276, "math_addToVariable"=4076863488, "math_addVToVariable"=4076863489, "math_subToVariable"=4076863490, "math_subVToVariable"=4076863491, "math_multToVariable"=4076863492, "math_multvToVariable"=4076863493, "math_divideToVariable"=4076863494, "math_divideVToVariable"=4076863495, "math_modToVariable"=4076863496, "math_modVToVariable"=4076863497, "logic_and"=4093640704, "logic_or"=4093640706, "logic_xor"=4093640708, "set_1Galvo"=101712113, "set_x-Galvo"=102760689, "set_y-Galvo"=103809265, "set_z-Fokus"=104857841, "set_1Galvo_position-only"=101711937, "set_x-Galvo_position-only"=102760513, "set_y-Galvo_position-only"=103809089, "set_z-Fokus_position-only"=104857665, "set_x-Galvo_position-only_ticket"=102764609, "set_y-Galvo_position-only_ticket"=103813185, "set_z-Fokus_position-only_ticket"=104861761, "set_x-Galvo_relativ-only"=102760577, "set_y-Galvo_relativ-only"=103809153, "set_z-Fokus_relativ-only"=104857729, "set_x-Galvo_speed-only"=102760481, "set_y-Galvo_speed-only"=103809057, "set_z-Fokus_speed-only"=104857633, "read_1Galvo_ticket"=101716032, "read_x-Galvo_ticket"=102764608, "read_y-Galvo_ticket"=103813184, "read_z-Focus_ticket"=104861760, "x-Galvo_pos_fromVar"=102760515, "y-Galvo_pos_fromVar"=103809091, "z-Focus_pos_fromVar"=104857667, "Servo0"=67108865, "Servo0-enable"=68091911, "Servo0-disable"=68091919, "Servo1"=68157441, "Servo1-enable"=69140487, "Servo1-disable"=69140495, "EnablePower0-SM"=2148466695, "DisablePower0-SM"=2148466703, "EnablePower1-Thermo1"=2149515271, "DisablePower1-Thermo1"=2149515279, "EnablePower2-Cam"=2150563847, "DisablePower2-Cam"=2150563855, "EnablePower3-Thermo2"=2151612423, "DisablePower3-Thermo2"=2151612431, "EnablePower4-Laser0"=2152660999, "DisablePower4-Laser0"=2152661007, "EnablePower5"=2153709575, "DisablePower5"=2153709583, "EnablePower6-Laser1"=2154758151, "DisablePower6-Laser1"=2154758159, "EnablePower7-SAM"=2155806727, "DisablePower7-SAM"=2155806735, "EnablePower8-Laser2"=2156855303, "DisablePower8-Laser2"=2156855311, "EnablePower9-TSM"=2157903879, "DisablePower9-TSM"=2157903887, "EnablePower10-Laser3"=2158952455, "DisablePower10-Laser3"=2158952463, "EnablePower11-Servo"=2160001031, "DisablePower11-Servo"=2160001039, "EnablePower12-Laser4"=2161049607, "DisablePower12-Laser4"=2161049615, "EnableSMPower2-DCC22"=2167341063, "DisableSMPower2-DCC22"=2167341071, "EnableSMPower3-6220"=2168389639, "DisableSMPower3-6220"=2168389647, "EnableSMPower4-6210"=2169438215, "DisableSMPower4-6210"=2169438223] ("command")
  w97 = 1  # 1 will be repeated
  w100 = 2  # Var
  w96 = -7  # commands in loop
  w101 = T4 4043379297 items=["read_x-Motor_status_ticket"=17305600, "init_x-Motor"=17760263, "read_x-Motor_absolute_ticket"=16781312, "move_x-Motor_absolute"=16777217, "move_x-Motor_relative"=16842753, "read_x-Motor_speed"=16977920, "set_x-Motor_speed"=16973825, "read_y-Motor_status_ticket"=18354176, "init_y-Motor"=18808839, "read_y-Motor_absolute_ticket"=17829888, "move_y-Motor_absolute"=17825793, "move_y-Motor_relative"=17891329, "read_y-Motor_speed"=18026496, "set_y-Motor_speed"=18022401, "read_z-Motor_status_ticket"=19402752, "init_z-Motor"=19857415, "stop_z-Motor"=19857423, "start_z-Motor"=19857422, "read_z-Motor_absolute_ticket"=18878464, "move_z-Motor_absolute"=18874369, "move_z-Motor_relative"=18939905, "read_Objective_status_ticket"=20451328, "init_Objective"=20905991, "read_Objective_absolute_ticket"=19927040, "move_Objective_absolute"=19922945, "move_Objective_relative"=19988481, "read_Objective-Motor_speed"=20123648, "set_Objective-Motor_speed"=20119553, "read_Filter_status_ticket"=21499904, "init_Filter"=21954567, "read_Filter_absolute_ticket"=20975616, "move_Filter_absolute"=20971521, "move_Filter_relative"=21037057, "read_Filter-Motor_speed"=21172224, "set_Filter-Motor_speed"=21168129, "read_Trans-Rad_status_ticket"=22548480, "init_Trans-Rad"=23003143, "read_Trans-Rad_absolute_ticket"=22024192, "move_Trans-Rad_absolute"=22020097, "move_Trans-Rad_relative"=22085633, "read_Trans-Motor_speed"=22220800, "set_Trans-Motor_speed"=22216705, "read_FRET_status_ticket"=23597056, "init_FRET"=24051719, "read_FRET_absolute_ticket"=23072768, "move_FRET_absolute"=23068673, "move_FRET_relative"=23134209, "read_FRET-Motor_speed"=23269376, "set_FRET-Motor_speed"=23265281, "read_SI-Rad_status_ticket"=24645632, "init_SI-Rad"=25100295, "read_SI-Rad_absolute_ticket"=24121344, "move_SI-Rad_absolute"=24117249, "move_SI-Rad_relative"=24182785, "read_SI-Rad_speed"=24317952, "set_SI-Rad_speed"=24313857, "end_no_ticket"=4027514895, "end_ticket"=4027518991, "IO-read_bank0"=3489665024, "IO-write_bank0"=3489660929, "IO-read_bank1"=3506442240, "IO-write_bank1"=3506438145, "DA0-0_LED365"=2684354561, "DA0-1_LED385"=2685403137, "DA0-2_LED440"=2686451713, "DA0-3_LED470"=2687500289, "DA0-4_LED510"=2688548865, "DA0-5_LED550"=2689597441, "DA0-6_LED590"=2690646017, "DA0-7_LED640"=2691694593, "DA1-0_LED-R"=2701131777, "DA1-1_LED-G"=2702180353, "DA1-2_LED-B"=2703228929, "DA1-3_LED-AF"=2704277505, "DA1-4"=2705326081, "DA1-5"=2706374657, "DA1-6"=2707423233, "DA1-7"=2708471809, "DA2-Laser0"=2717908993, "DA2-Laser1"=2718957569, "DA2-Laser2"=2720006145, "DA2-Laser3"=2721054721, "DA2-Laser4"=2722103297, "Analog-read_AD0-0"=2818576384, "Analog-read-store_AD0-0"=2818572290, "IO-delay_bank0"=3489923073, "IO-delay_bank0_fromVar"=3489923075, "read_cam_clock"=3289124864, "store_cam_clock"=3289120770, "read_cam_phase"=3289190400, "store_cam_phase"=3289190402, "Read ticks"=4027518976, "Read ticks to var"=4027518978, "Read IP"=4043313152, "Read IP into var"=4043313154, "Set IP from var"=4043309059, "Set IP from var, relative"=4043313155, "decrement_branchRel_if_equal"=4043374945, "decrement_branchRel_if_greaterequal"=4043375201, "decrement_branchRel_if_greaterequal_withTicket"=4043379297, "decrement_branchRel_if_smaller"=4043375457, "increment_branchRel_if_smaller"=4043375473, "readVar"=4060090368, "writeVar"=4060086273, "readVar_and_copy_to_var2"=4060086275, "loadVar2_andcopy_var1"=4060086276, "math_addToVariable"=4076863488, "math_addVToVariable"=4076863489, "math_subToVariable"=4076863490, "math_subVToVariable"=4076863491, "math_multToVariable"=4076863492, "math_multvToVariable"=4076863493, "math_divideToVariable"=4076863494, "math_divideVToVariable"=4076863495, "math_modToVariable"=4076863496, "math_modVToVariable"=4076863497, "logic_and"=4093640704, "logic_or"=4093640706, "logic_xor"=4093640708, "set_1Galvo"=101712113, "set_x-Galvo"=102760689, "set_y-Galvo"=103809265, "set_z-Fokus"=104857841, "set_1Galvo_position-only"=101711937, "set_x-Galvo_position-only"=102760513, "set_y-Galvo_position-only"=103809089, "set_z-Fokus_position-only"=104857665, "set_x-Galvo_position-only_ticket"=102764609, "set_y-Galvo_position-only_ticket"=103813185, "set_z-Fokus_position-only_ticket"=104861761, "set_x-Galvo_relativ-only"=102760577, "set_y-Galvo_relativ-only"=103809153, "set_z-Fokus_relativ-only"=104857729, "set_x-Galvo_speed-only"=102760481, "set_y-Galvo_speed-only"=103809057, "set_z-Fokus_speed-only"=104857633, "read_1Galvo_ticket"=101716032, "read_x-Galvo_ticket"=102764608, "read_y-Galvo_ticket"=103813184, "read_z-Focus_ticket"=104861760, "x-Galvo_pos_fromVar"=102760515, "y-Galvo_pos_fromVar"=103809091, "z-Focus_pos_fromVar"=104857667, "Servo0"=67108865, "Servo0-enable"=68091911, "Servo0-disable"=68091919, "Servo1"=68157441, "Servo1-enable"=69140487, "Servo1-disable"=69140495, "EnablePower0-SM"=2148466695, "DisablePower0-SM"=2148466703, "EnablePower1-Thermo1"=2149515271, "DisablePower1-Thermo1"=2149515279, "EnablePower2-Cam"=2150563847, "DisablePower2-Cam"=2150563855, "EnablePower3-Thermo2"=2151612423, "DisablePower3-Thermo2"=2151612431, "EnablePower4-Laser0"=2152660999, "DisablePower4-Laser0"=2152661007, "EnablePower5"=2153709575, "DisablePower5"=2153709583, "EnablePower6-Laser1"=2154758151, "DisablePower6-Laser1"=2154758159, "EnablePower7-SAM"=2155806727, "DisablePower7-SAM"=2155806735, "EnablePower8-Laser2"=2156855303, "DisablePower8-Laser2"=2156855311, "EnablePower9-TSM"=2157903879, "DisablePower9-TSM"=2157903887, "EnablePower10-Laser3"=2158952455, "DisablePower10-Laser3"=2158952463, "EnablePower11-Servo"=2160001031, "DisablePower11-Servo"=2160001039, "EnablePower12-Laser4"=2161049607, "DisablePower12-Laser4"=2161049615, "EnableSMPower2-DCC22"=2167341063, "DisableSMPower2-DCC22"=2167341071, "EnableSMPower3-6220"=2168389639, "DisableSMPower3-6220"=2168389647, "EnableSMPower4-6210"=2169438215, "DisableSMPower4-6210"=2169438223] ("command")
  w102 = u32 2  # 2*0.5 turntimes
  w111 = T4 3489660929 items=["read_x-Motor_status_ticket"=17305600, "init_x-Motor"=17760263, "read_x-Motor_absolute_ticket"=16781312, "move_x-Motor_absolute"=16777217, "move_x-Motor_relative"=16842753, "read_y-Motor_status_ticket"=18354176, "init_y-Motor"=18808839, "read_y-Motor_absolute_ticket"=17829888, "move_y-Motor_absolute"=17825793, "move_y-Motor_relative"=17891329, "read_z-Motor_status_ticket"=19402752, "init_z-Motor"=19857415, "stop_z-Motor"=19857423, "start_z-Motor"=19857422, "read_z-Motor_absolute_ticket"=18878464, "move_z-Motor_absolute"=18874369, "move_z-Motor_relative"=18939905, "end_no_ticket"=4027514895, "end_ticket"=4027518991, "IO-read_bank0"=3489665024, "IO-write_bank0"=3489660929, "IO-read_bank1"=3506442240, "IO-write_bank1"=3506438145, "IO-delay_bank0"=3489923073, "IO-delay_bank0_fromVar"=3489923075, "read_cam_clock"=3289124864, "store_cam_clock"=3289120770, "read_cam_phase"=3289190400, "set_cam_deadtime"=3288989697, "set_cam_10uscycles"=3289055233, "set_cam_10uscycles_fromVariable"=3289055235, "calc_cam"=3289317386, "store_cam_Var"=3289251842, "math_addToVariable"=4060086278, "readVar"=4060090368, "writeVar"=4060086273, "copyVar"=4060086276, "decrement_branchRel_if_equal"=4043374945, "decrement_branchRel_if_greaterequal"=4043375201, "decrement_branchRel_if_greaterequal_withTicket"=4043379297, "decrement_branchRel_if_smaller"=4043375457, "increment_branchRel_if_smaller"=4043375473, "set_x-Galvo"=1612710129, "set_y-Galvo"=1613758705, "set_z-Fokus"=1614807281, "set_x-Galvo_position-only"=1612709953, "set_y-Galvo_position-only"=1613758529, "set_z-Fokus_position-only"=1614807105, "set_x-Galvo_position-only_ticket"=1612714049, "set_y-Galvo_position-only_ticket"=1613762625, "set_z-Fokus_position-only_ticket"=1614811201, "read_x-Galvo_ticket"=1612714048, "read_y-Galvo_ticket"=1613762624, "read_z-Focus_ticket"=1614811200, "x-Galvo_pos_fromVar"=1612709955, "y-Galvo_pos_fromVar"=1613758531, "z-Focus_pos_fromVar"=1614807107] ("command")
  w126 = 2  # Var2 linecounter (subframe)
  w128 = T4 4060086273 items=["read_x-Motor_status_ticket"=17305600, "init_x-Motor"=17760263, "read_x-Motor_absolute_ticket"=16781312, "move_x-Motor_absolute"=16777217, "move_x-Motor_relative"=16842753, "read_x-Motor_speed"=16977920, "set_x-Motor_speed"=16973825, "read_y-Motor_status_ticket"=18354176, "init_y-Motor"=18808839, "read_y-Motor_absolute_ticket"=17829888, "move_y-Motor_absolute"=17825793, "move_y-Motor_relative"=17891329, "read_y-Motor_speed"=18026496, "set_y-Motor_speed"=18022401, "read_z-Motor_status_ticket"=19402752, "init_z-Motor"=19857415, "stop_z-Motor"=19857423, "start_z-Motor"=19857422, "read_z-Motor_absolute_ticket"=18878464, "move_z-Motor_absolute"=18874369, "move_z-Motor_relative"=18939905, "read_Objective_status_ticket"=20451328, "init_Objective"=20905991, "read_Objective_absolute_ticket"=19927040, "move_Objective_absolute"=19922945, "move_Objective_relative"=19988481, "read_Objective-Motor_speed"=20123648, "set_Objective-Motor_speed"=20119553, "read_Filter_status_ticket"=21499904, "init_Filter"=21954567, "read_Filter_absolute_ticket"=20975616, "move_Filter_absolute"=20971521, "move_Filter_relative"=21037057, "read_Filter-Motor_speed"=21172224, "set_Filter-Motor_speed"=21168129, "read_Trans-Rad_status_ticket"=22548480, "init_Trans-Rad"=23003143, "read_Trans-Rad_absolute_ticket"=22024192, "move_Trans-Rad_absolute"=22020097, "move_Trans-Rad_relative"=22085633, "read_Trans-Motor_speed"=22220800, "set_Trans-Motor_speed"=22216705, "read_FRET_status_ticket"=23597056, "init_FRET"=24051719, "read_FRET_absolute_ticket"=23072768, "move_FRET_absolute"=23068673, "move_FRET_relative"=23134209, "read_FRET-Motor_speed"=23269376, "set_FRET-Motor_speed"=23265281, "read_SI-Rad_status_ticket"=24645632, "init_SI-Rad"=25100295, "read_SI-Rad_absolute_ticket"=24121344, "move_SI-Rad_absolute"=24117249, "move_SI-Rad_relative"=24182785, "read_SI-Rad_speed"=24317952, "set_SI-Rad_speed"=24313857, "end_no_ticket"=4027514895, "end_ticket"=4027518991, "IO-read_bank0"=3489665024, "IO-write_bank0"=3489660929, "IO-read_bank1"=3506442240, "IO-write_bank1"=3506438145, "DA0-0_LED365"=2684354561, "DA0-1_LED385"=2685403137, "DA0-2_LED440"=2686451713, "DA0-3_LED470"=2687500289, "DA0-4_LED510"=2688548865, "DA0-5_LED550"=2689597441, "DA0-6_LED590"=2690646017, "DA0-7_LED640"=2691694593, "DA1-0_LED-R"=2701131777, "DA1-1_LED-G"=2702180353, "DA1-2_LED-B"=2703228929, "DA1-3_LED-AF"=2704277505, "DA1-4"=2705326081, "DA1-5"=2706374657, "DA1-6"=2707423233, "DA1-7"=2708471809, "DA2-Laser0"=2717908993, "DA2-Laser1"=2718957569, "DA2-Laser2"=2720006145, "DA2-Laser3"=2721054721, "DA2-Laser4"=2722103297, "Analog-read_AD0-0"=2818576384, "Analog-read-store_AD0-0"=2818572290, "IO-delay_bank0"=3489923073, "IO-delay_bank0_fromVar"=3489923075, "read_cam_clock"=3289124864, "store_cam_clock"=3289120770, "read_cam_phase"=3289190400, "store_cam_phase"=3289190402, "Read ticks"=4027518976, "Read ticks to var"=4027518978, "Read IP"=4043313152, "Read IP into var"=4043313154, "Set IP from var"=4043309059, "Set IP from var, relative"=4043313155, "decrement_branchRel_if_equal"=4043374945, "decrement_branchRel_if_greaterequal"=4043375201, "decrement_branchRel_if_greaterequal_withTicket"=4043379297, "decrement_branchRel_if_smaller"=4043375457, "increment_branchRel_if_smaller"=4043375473, "readVar"=4060090368, "writeVar"=4060086273, "readVar_and_copy_to_var2"=4060086275, "loadVar2_andcopy_var1"=4060086276, "math_addToVariable"=4076863488, "math_addVToVariable"=4076863489, "math_subToVariable"=4076863490, "math_subVToVariable"=4076863491, "math_multToVariable"=4076863492, "math_multvToVariable"=4076863493, "math_divideToVariable"=4076863494, "math_divideVToVariable"=4076863495, "math_modToVariable"=4076863496, "math_modVToVariable"=4076863497, "logic_and"=4093640704, "logic_or"=4093640706, "logic_xor"=4093640708, "set_1Galvo"=101712113, "set_x-Galvo"=102760689, "set_y-Galvo"=103809265, "set_z-Fokus"=104857841, "set_1Galvo_position-only"=101711937, "set_x-Galvo_position-only"=102760513, "set_y-Galvo_position-only"=103809089, "set_z-Fokus_position-only"=104857665, "set_x-Galvo_position-only_ticket"=102764609, "set_y-Galvo_position-only_ticket"=103813185, "set_z-Fokus_position-only_ticket"=104861761, "set_x-Galvo_relativ-only"=102760577, "set_y-Galvo_relativ-only"=103809153, "set_z-Fokus_relativ-only"=104857729, "set_x-Galvo_speed-only"=102760481, "set_y-Galvo_speed-only"=103809057, "set_z-Fokus_speed-only"=104857633, "read_1Galvo_ticket"=101716032, "read_x-Galvo_ticket"=102764608, "read_y-Galvo_ticket"=103813184, "read_z-Focus_ticket"=104861760, "x-Galvo_pos_fromVar"=102760515, "y-Galvo_pos_fromVar"=103809091, "z-Focus_pos_fromVar"=104857667, "Servo0"=67108865, "Servo0-enable"=68091911, "Servo0-disable"=68091919, "Servo1"=68157441, "Servo1-enable"=69140487, "Servo1-disable"=69140495, "EnablePower0-SM"=2148466695, "DisablePower0-SM"=2148466703, "EnablePower1-Thermo1"=2149515271, "DisablePower1-Thermo1"=2149515279, "EnablePower2-Cam"=2150563847, "DisablePower2-Cam"=2150563855, "EnablePower3-Thermo2"=2151612423, "DisablePower3-Thermo2"=2151612431, "EnablePower4-Laser0"=2152660999, "DisablePower4-Laser0"=2152661007, "EnablePower5"=2153709575, "DisablePower5"=2153709583, "EnablePower6-Laser1"=2154758151, "DisablePower6-Laser1"=2154758159, "EnablePower7-SAM"=2155806727, "DisablePower7-SAM"=2155806735, "EnablePower8-Laser2"=2156855303, "DisablePower8-Laser2"=2156855311, "EnablePower9-TSM"=2157903879, "DisablePower9-TSM"=2157903887, "EnablePower10-Laser3"=2158952455, "DisablePower10-Laser3"=2158952463, "EnablePower11-Servo"=2160001031, "DisablePower11-Servo"=2160001039, "EnablePower12-Laser4"=2161049607, "DisablePower12-Laser4"=2161049615, "EnableSMPower2-DCC22"=2167341063, "DisableSMPower2-DCC22"=2167341071, "EnableSMPower3-6220"=2168389639, "DisableSMPower3-6220"=2168389647, "EnableSMPower4-6210"=2169438215, "DisableSMPower4-6210"=2169438223] ("command")
  w138 = 10.0  # µs
  w145 = 123456789.0  # no speedlimit
  w154 = 1  # 1 will be repeated
  w157 = 3  # Var
  w158 = -6  # commands in loop
  w159 = T4 4043379297 items=["read_x-Motor_status_ticket"=17305600, "init_x-Motor"=17760263, "read_x-Motor_absolute_ticket"=16781312, "move_x-Motor_absolute"=16777217, "move_x-Motor_relative"=16842753, "read_x-Motor_speed"=16977920, "set_x-Motor_speed"=16973825, "read_y-Motor_status_ticket"=18354176, "init_y-Motor"=18808839, "read_y-Motor_absolute_ticket"=17829888, "move_y-Motor_absolute"=17825793, "move_y-Motor_relative"=17891329, "read_y-Motor_speed"=18026496, "set_y-Motor_speed"=18022401, "read_z-Motor_status_ticket"=19402752, "init_z-Motor"=19857415, "stop_z-Motor"=19857423, "start_z-Motor"=19857422, "read_z-Motor_absolute_ticket"=18878464, "move_z-Motor_absolute"=18874369, "move_z-Motor_relative"=18939905, "read_Objective_status_ticket"=20451328, "init_Objective"=20905991, "read_Objective_absolute_ticket"=19927040, "move_Objective_absolute"=19922945, "move_Objective_relative"=19988481, "read_Objective-Motor_speed"=20123648, "set_Objective-Motor_speed"=20119553, "read_Filter_status_ticket"=21499904, "init_Filter"=21954567, "read_Filter_absolute_ticket"=20975616, "move_Filter_absolute"=20971521, "move_Filter_relative"=21037057, "read_Filter-Motor_speed"=21172224, "set_Filter-Motor_speed"=21168129, "read_Trans-Rad_status_ticket"=22548480, "init_Trans-Rad"=23003143, "read_Trans-Rad_absolute_ticket"=22024192, "move_Trans-Rad_absolute"=22020097, "move_Trans-Rad_relative"=22085633, "read_Trans-Motor_speed"=22220800, "set_Trans-Motor_speed"=22216705, "read_FRET_status_ticket"=23597056, "init_FRET"=24051719, "read_FRET_absolute_ticket"=23072768, "move_FRET_absolute"=23068673, "move_FRET_relative"=23134209, "read_FRET-Motor_speed"=23269376, "set_FRET-Motor_speed"=23265281, "read_SI-Rad_status_ticket"=24645632, "init_SI-Rad"=25100295, "read_SI-Rad_absolute_ticket"=24121344, "move_SI-Rad_absolute"=24117249, "move_SI-Rad_relative"=24182785, "read_SI-Rad_speed"=24317952, "set_SI-Rad_speed"=24313857, "end_no_ticket"=4027514895, "end_ticket"=4027518991, "IO-read_bank0"=3489665024, "IO-write_bank0"=3489660929, "IO-read_bank1"=3506442240, "IO-write_bank1"=3506438145, "DA0-0_LED365"=2684354561, "DA0-1_LED385"=2685403137, "DA0-2_LED440"=2686451713, "DA0-3_LED470"=2687500289, "DA0-4_LED510"=2688548865, "DA0-5_LED550"=2689597441, "DA0-6_LED590"=2690646017, "DA0-7_LED640"=2691694593, "DA1-0_LED-R"=2701131777, "DA1-1_LED-G"=2702180353, "DA1-2_LED-B"=2703228929, "DA1-3_LED-AF"=2704277505, "DA1-4"=2705326081, "DA1-5"=2706374657, "DA1-6"=2707423233, "DA1-7"=2708471809, "DA2-Laser0"=2717908993, "DA2-Laser1"=2718957569, "DA2-Laser2"=2720006145, "DA2-Laser3"=2721054721, "DA2-Laser4"=2722103297, "Analog-read_AD0-0"=2818576384, "Analog-read-store_AD0-0"=2818572290, "IO-delay_bank0"=3489923073, "IO-delay_bank0_fromVar"=3489923075, "read_cam_clock"=3289124864, "store_cam_clock"=3289120770, "read_cam_phase"=3289190400, "store_cam_phase"=3289190402, "Read ticks"=4027518976, "Read ticks to var"=4027518978, "Read IP"=4043313152, "Read IP into var"=4043313154, "Set IP from var"=4043309059, "Set IP from var, relative"=4043313155, "decrement_branchRel_if_equal"=4043374945, "decrement_branchRel_if_greaterequal"=4043375201, "decrement_branchRel_if_greaterequal_withTicket"=4043379297, "decrement_branchRel_if_smaller"=4043375457, "increment_branchRel_if_smaller"=4043375473, "readVar"=4060090368, "writeVar"=4060086273, "readVar_and_copy_to_var2"=4060086275, "loadVar2_andcopy_var1"=4060086276, "math_addToVariable"=4076863488, "math_addVToVariable"=4076863489, "math_subToVariable"=4076863490, "math_subVToVariable"=4076863491, "math_multToVariable"=4076863492, "math_multvToVariable"=4076863493, "math_divideToVariable"=4076863494, "math_divideVToVariable"=4076863495, "math_modToVariable"=4076863496, "math_modVToVariable"=4076863497, "logic_and"=4093640704, "logic_or"=4093640706, "logic_xor"=4093640708, "set_1Galvo"=101712113, "set_x-Galvo"=102760689, "set_y-Galvo"=103809265, "set_z-Fokus"=104857841, "set_1Galvo_position-only"=101711937, "set_x-Galvo_position-only"=102760513, "set_y-Galvo_position-only"=103809089, "set_z-Fokus_position-only"=104857665, "set_x-Galvo_position-only_ticket"=102764609, "set_y-Galvo_position-only_ticket"=103813185, "set_z-Fokus_position-only_ticket"=104861761, "set_x-Galvo_relativ-only"=102760577, "set_y-Galvo_relativ-only"=103809153, "set_z-Fokus_relativ-only"=104857729, "set_x-Galvo_speed-only"=102760481, "set_y-Galvo_speed-only"=103809057, "set_z-Fokus_speed-only"=104857633, "read_1Galvo_ticket"=101716032, "read_x-Galvo_ticket"=102764608, "read_y-Galvo_ticket"=103813184, "read_z-Focus_ticket"=104861760, "x-Galvo_pos_fromVar"=102760515, "y-Galvo_pos_fromVar"=103809091, "z-Focus_pos_fromVar"=104857667, "Servo0"=67108865, "Servo0-enable"=68091911, "Servo0-disable"=68091919, "Servo1"=68157441, "Servo1-enable"=69140487, "Servo1-disable"=69140495, "EnablePower0-SM"=2148466695, "DisablePower0-SM"=2148466703, "EnablePower1-Thermo1"=2149515271, "DisablePower1-Thermo1"=2149515279, "EnablePower2-Cam"=2150563847, "DisablePower2-Cam"=2150563855, "EnablePower3-Thermo2"=2151612423, "DisablePower3-Thermo2"=2151612431, "EnablePower4-Laser0"=2152660999, "DisablePower4-Laser0"=2152661007, "EnablePower5"=2153709575, "DisablePower5"=2153709583, "EnablePower6-Laser1"=2154758151, "DisablePower6-Laser1"=2154758159, "EnablePower7-SAM"=2155806727, "DisablePower7-SAM"=2155806735, "EnablePower8-Laser2"=2156855303, "DisablePower8-Laser2"=2156855311, "EnablePower9-TSM"=2157903879, "DisablePower9-TSM"=2157903887, "EnablePower10-Laser3"=2158952455, "DisablePower10-Laser3"=2158952463, "EnablePower11-Servo"=2160001031, "DisablePower11-Servo"=2160001039, "EnablePower12-Laser4"=2161049607, "DisablePower12-Laser4"=2161049615, "EnableSMPower2-DCC22"=2167341063, "DisableSMPower2-DCC22"=2167341071, "EnableSMPower3-6220"=2168389639, "DisableSMPower3-6220"=2168389647, "EnableSMPower4-6210"=2169438215, "DisableSMPower4-6210"=2169438223] ("command")
  w160 = 3  # Var3  framecounter
  w162 = T4 4060086273 items=["read_x-Motor_status_ticket"=17305600, "init_x-Motor"=17760263, "read_x-Motor_absolute_ticket"=16781312, "move_x-Motor_absolute"=16777217, "move_x-Motor_relative"=16842753, "read_x-Motor_speed"=16977920, "set_x-Motor_speed"=16973825, "read_y-Motor_status_ticket"=18354176, "init_y-Motor"=18808839, "read_y-Motor_absolute_ticket"=17829888, "move_y-Motor_absolute"=17825793, "move_y-Motor_relative"=17891329, "read_y-Motor_speed"=18026496, "set_y-Motor_speed"=18022401, "read_z-Motor_status_ticket"=19402752, "init_z-Motor"=19857415, "stop_z-Motor"=19857423, "start_z-Motor"=19857422, "read_z-Motor_absolute_ticket"=18878464, "move_z-Motor_absolute"=18874369, "move_z-Motor_relative"=18939905, "read_Objective_status_ticket"=20451328, "init_Objective"=20905991, "read_Objective_absolute_ticket"=19927040, "move_Objective_absolute"=19922945, "move_Objective_relative"=19988481, "read_Objective-Motor_speed"=20123648, "set_Objective-Motor_speed"=20119553, "read_Filter_status_ticket"=21499904, "init_Filter"=21954567, "read_Filter_absolute_ticket"=20975616, "move_Filter_absolute"=20971521, "move_Filter_relative"=21037057, "read_Filter-Motor_speed"=21172224, "set_Filter-Motor_speed"=21168129, "read_Trans-Rad_status_ticket"=22548480, "init_Trans-Rad"=23003143, "read_Trans-Rad_absolute_ticket"=22024192, "move_Trans-Rad_absolute"=22020097, "move_Trans-Rad_relative"=22085633, "read_Trans-Motor_speed"=22220800, "set_Trans-Motor_speed"=22216705, "read_FRET_status_ticket"=23597056, "init_FRET"=24051719, "read_FRET_absolute_ticket"=23072768, "move_FRET_absolute"=23068673, "move_FRET_relative"=23134209, "read_FRET-Motor_speed"=23269376, "set_FRET-Motor_speed"=23265281, "read_SI-Rad_status_ticket"=24645632, "init_SI-Rad"=25100295, "read_SI-Rad_absolute_ticket"=24121344, "move_SI-Rad_absolute"=24117249, "move_SI-Rad_relative"=24182785, "read_SI-Rad_speed"=24317952, "set_SI-Rad_speed"=24313857, "end_no_ticket"=4027514895, "end_ticket"=4027518991, "IO-read_bank0"=3489665024, "IO-write_bank0"=3489660929, "IO-read_bank1"=3506442240, "IO-write_bank1"=3506438145, "DA0-0_LED365"=2684354561, "DA0-1_LED385"=2685403137, "DA0-2_LED440"=2686451713, "DA0-3_LED470"=2687500289, "DA0-4_LED510"=2688548865, "DA0-5_LED550"=2689597441, "DA0-6_LED590"=2690646017, "DA0-7_LED640"=2691694593, "DA1-0_LED-R"=2701131777, "DA1-1_LED-G"=2702180353, "DA1-2_LED-B"=2703228929, "DA1-3_LED-AF"=2704277505, "DA1-4"=2705326081, "DA1-5"=2706374657, "DA1-6"=2707423233, "DA1-7"=2708471809, "DA2-Laser0"=2717908993, "DA2-Laser1"=2718957569, "DA2-Laser2"=2720006145, "DA2-Laser3"=2721054721, "DA2-Laser4"=2722103297, "Analog-read_AD0-0"=2818576384, "Analog-read-store_AD0-0"=2818572290, "IO-delay_bank0"=3489923073, "IO-delay_bank0_fromVar"=3489923075, "read_cam_clock"=3289124864, "store_cam_clock"=3289120770, "read_cam_phase"=3289190400, "store_cam_phase"=3289190402, "Read ticks"=4027518976, "Read ticks to var"=4027518978, "Read IP"=4043313152, "Read IP into var"=4043313154, "Set IP from var"=4043309059, "Set IP from var, relative"=4043313155, "decrement_branchRel_if_equal"=4043374945, "decrement_branchRel_if_greaterequal"=4043375201, "decrement_branchRel_if_greaterequal_withTicket"=4043379297, "decrement_branchRel_if_smaller"=4043375457, "increment_branchRel_if_smaller"=4043375473, "readVar"=4060090368, "writeVar"=4060086273, "readVar_and_copy_to_var2"=4060086275, "loadVar2_andcopy_var1"=4060086276, "math_addToVariable"=4076863488, "math_addVToVariable"=4076863489, "math_subToVariable"=4076863490, "math_subVToVariable"=4076863491, "math_multToVariable"=4076863492, "math_multvToVariable"=4076863493, "math_divideToVariable"=4076863494, "math_divideVToVariable"=4076863495, "math_modToVariable"=4076863496, "math_modVToVariable"=4076863497, "logic_and"=4093640704, "logic_or"=4093640706, "logic_xor"=4093640708, "set_1Galvo"=101712113, "set_x-Galvo"=102760689, "set_y-Galvo"=103809265, "set_z-Fokus"=104857841, "set_1Galvo_position-only"=101711937, "set_x-Galvo_position-only"=102760513, "set_y-Galvo_position-only"=103809089, "set_z-Fokus_position-only"=104857665, "set_x-Galvo_position-only_ticket"=102764609, "set_y-Galvo_position-only_ticket"=103813185, "set_z-Fokus_position-only_ticket"=104861761, "set_x-Galvo_relativ-only"=102760577, "set_y-Galvo_relativ-only"=103809153, "set_z-Fokus_relativ-only"=104857729, "set_x-Galvo_speed-only"=102760481, "set_y-Galvo_speed-only"=103809057, "set_z-Fokus_speed-only"=104857633, "read_1Galvo_ticket"=101716032, "read_x-Galvo_ticket"=102764608, "read_y-Galvo_ticket"=103813184, "read_z-Focus_ticket"=104861760, "x-Galvo_pos_fromVar"=102760515, "y-Galvo_pos_fromVar"=103809091, "z-Focus_pos_fromVar"=104857667, "Servo0"=67108865, "Servo0-enable"=68091911, "Servo0-disable"=68091919, "Servo1"=68157441, "Servo1-enable"=69140487, "Servo1-disable"=69140495, "EnablePower0-SM"=2148466695, "DisablePower0-SM"=2148466703, "EnablePower1-Thermo1"=2149515271, "DisablePower1-Thermo1"=2149515279, "EnablePower2-Cam"=2150563847, "DisablePower2-Cam"=2150563855, "EnablePower3-Thermo2"=2151612423, "DisablePower3-Thermo2"=2151612431, "EnablePower4-Laser0"=2152660999, "DisablePower4-Laser0"=2152661007, "EnablePower5"=2153709575, "DisablePower5"=2153709583, "EnablePower6-Laser1"=2154758151, "DisablePower6-Laser1"=2154758159, "EnablePower7-SAM"=2155806727, "DisablePower7-SAM"=2155806735, "EnablePower8-Laser2"=2156855303, "DisablePower8-Laser2"=2156855311, "EnablePower9-TSM"=2157903879, "DisablePower9-TSM"=2157903887, "EnablePower10-Laser3"=2158952455, "DisablePower10-Laser3"=2158952463, "EnablePower11-Servo"=2160001031, "DisablePower11-Servo"=2160001039, "EnablePower12-Laser4"=2161049607, "DisablePower12-Laser4"=2161049615, "EnableSMPower2-DCC22"=2167341063, "DisableSMPower2-DCC22"=2167341071, "EnableSMPower3-6220"=2168389639, "DisableSMPower3-6220"=2168389647, "EnableSMPower4-6210"=2169438215, "DisableSMPower4-6210"=2169438223] ("command")
  w170 = 2  # nm/count
  w190 = T4 4027518991 items=["read_x-Motor_status_ticket"=17305600, "init_x-Motor"=17760263, "read_x-Motor_absolute_ticket"=16781312, "move_x-Motor_absolute"=16777217, "move_x-Motor_relative"=16842753, "read_y-Motor_status_ticket"=18354176, "init_y-Motor"=18808839, "read_y-Motor_absolute_ticket"=17829888, "move_y-Motor_absolute"=17825793, "move_y-Motor_relative"=17891329, "read_z-Motor_status_ticket"=19402752, "init_z-Motor"=19857415, "stop_z-Motor"=19857423, "start_z-Motor"=19857422, "read_z-Motor_absolute_ticket"=18878464, "move_z-Motor_absolute"=18874369, "move_z-Motor_relative"=18939905, "end_no_ticket"=4027514895, "end_ticket"=4027518991, "IO-read_bank0"=3489665024, "IO-write_bank0"=3489660929, "IO-read_bank1"=3506442240, "IO-write_bank1"=3506438145, "IO-delay_bank0"=3489923073, "IO-delay_bank0_fromVar"=3489923075, "read_cam_clock"=3289124864, "store_cam_clock"=3289120770, "read_cam_phase"=3289190400, "set_cam_deadtime"=3288989697, "set_cam_10uscycles"=3289055233, "set_cam_10uscycles_fromVariable"=3289055235, "calc_cam"=3289317386, "store_cam_Var"=3289251842, "math_addToVariable"=4060086278, "readVar"=4060090368, "writeVar"=4060086273, "copyVar"=4060086276, "decrement_branchRel_if_equal"=4043374945, "decrement_branchRel_if_greaterequal"=4043375201, "decrement_branchRel_if_greaterequal_withTicket"=4043379297, "decrement_branchRel_if_smaller"=4043375457, "increment_branchRel_if_smaller"=4043375473, "set_x-Galvo"=1612710129, "set_y-Galvo"=1613758705, "set_z-Fokus"=1614807281, "set_x-Galvo_position-only"=1612709953, "set_y-Galvo_position-only"=1613758529, "set_z-Fokus_position-only"=1614807105, "set_x-Galvo_position-only_ticket"=1612714049, "set_y-Galvo_position-only_ticket"=1613762625, "set_z-Fokus_position-only_ticket"=1614811201, "read_x-Galvo_ticket"=1612714048, "read_y-Galvo_ticket"=1613762624, "read_z-Focus_ticket"=1614811200, "x-Galvo_pos_fromVar"=1612709955, "y-Galvo_pos_fromVar"=1613758531, "z-Focus_pos_fromVar"=1614807107] ("command")
  # "order is rel,abs,inc,incinc!"
  # "check if cam clock is ok!"
  # "bis hier etwa OK"
  # "fehlt relativ offset in var10"
  # "PhaseTurn"
  # "galvo turn"
  # "repeat modulo"
  # "fehlt relativ offset in var10"
  # "galvo start pos"
  # "wobbler start pos"
  # "start position\n0.5 RS above"
  # "a parabolic move:\nx=a/2 *t(t-1)+v*t"
  # "go back at end"
  n1 = Unbundle By Name("Constants") -> ("RollingShutter height- Pix"=w86:u16, "GalvoX-Blanking"=w168:dbl, "Wobbel-total"=w95:dbl, "WobbelAccel"=w142:dbl, "galvoxAccel"=w141:dbl, "Camera-StartLine"=w73:u32, "Camera-Endline"=w74:u32, "galvox-Line0"=w134:i16, "galvox-count/pix"=w77:dbl, "SCMOS-LineSpeed [10µs]"=w69:dbl, "SM_ticks"=w54:u32)  [unwired: 1 out]
  n2 = Unbundle By Name("User") -> ("z-distance_nm"=w169:i32, "#planes"=w146:u16, "NoOfPhaseImages"=w84:u16)
  n3 = Divide(x=w86, y=u16 2) -> (x/y=w75:dbl)
  n4 = Subtract(x=w73, y=w75) -> (x-y=w71:dbl)
  n5 = Add(x=w74, y=w75) -> (x+y=w72:dbl)
  n6 = Unbundle By Name("Constants") -> ("Camera-Endline"=w106:u32, "Trigger_ticks"=w48:u32, "RollingShutter height- Pix"=w85:u16)  [unwired: 3 out]
  n7 = Divide(x=w77, y=w69) -> (x/y=w36:dbl)
  "x vel" <- w36
  n8 = Increment(x=w72) -> (x+1=w65:dbl)
  n9 = Multiply(x=w71, y=w77) -> (x*y=w136:dbl)
  n10 = Multiply(x=w72, y=w77) -> (x*y=w135:dbl)
  n11 = Subtract "MovedPix"(x=w65, y=w71) -> (x-y=w70:dbl)
  n12 = Add(x=w135, y=w134) -> (x+y=w133:dbl)
  "xgalvoend" <- w133
  n13 = Add(x=w136, y=w134) -> (x+y=w76:dbl)
  "xgalvostart" <- w76
  n14 = Multiply "CamTicks"(x=w70, y=w69) -> (x*y=w68:dbl)
  n15 = Divide(x=w95, y=w84) -> (x/y=w30:dbl)
  "WobShift" <- w30
  n16 = Round Toward +Infinity(x=w68) -> (ceil(x): smallest int >= x=w67:dbl)
  n17 = Subtract(x=w76, y=w133) -> (x-y=w132:dbl)
  "~x-move" <- w132
  n18 = To Unsigned Long Integer "Cam-Ticks"(number=w67) -> (unsigned 32bit integer=w3:u32)
  "CamTics" <- w3
  n19 = Add(x=w106, y=w85) -> ()  [unwired: 1 out]
  n20 = call "MoveTime.vi"("maxaccel"=w142, "maxspeed"=w145, "dist"=w30) -> ("expected duration"=w144:dbl)
  "expected  Wduration" <- w144
  n21 = call "MoveTime.vi"("maxaccel"=w141, "maxspeed"=w145, "dist"=w132) -> ("expected duration"=w143:dbl)
  "expected xduration" <- w143
  n22 = Max & Min(x=w144, y=w143) -> (max(x,y)=w130:dbl)  [unwired: 1 out]
  n23 = Multiply(x=w36, y=w3) -> (x*y=w37:dbl)
  "GalvoMove" <- w37
  n24 = Divide(x=w130, y=u32 2) -> (x/y=w131:dbl)
  n25 = To Unsigned Long Integer(number=w131) -> (unsigned 32bit integer=w21:u32)
  "Half Turn_ticks" <- w21
  n26 = Compound Arithmetic op=ADD(w21, w21, w54, u32 1 ("value")) -> (w50:u32)
  "PredictionTime" <- w50
  n27 = Compound Arithmetic op=ADD(w21, w21, w3) -> (w51:u32)
  "FrameClock" <- w51
  n28 = Multiply(x=0.0, y=w138) -> (x*y=w139:dbl)
  n29 = formula code="a=(-x-2*v*t)/(t*(t-1));"("x"=w37, "v"=w36, "t"=w21) -> ("a"=w35:dbl)
  "galvo a" <- w35
  n30 = formula code="a=x/(t*(t-1));"("x"=w30, "t"=w21) -> ("a"=w31:dbl)
  "phase a" <- w31
  n31 = Multiply(x=w146, y=w84) -> (x*y=w167:u16)
  n32 = Bundle By Name(cluster=T1 {"Camera-Exposure"=550.5, "CameraImages"=245} ("Cluster"), "Camera-Exposure"=w139, "CameraImages"=w167) -> (→"Camera":T1)
  n33 = call "SIAM-TMSI.vi"("Type"=enum8{"acc", "vel", "abs", "offset"}."offset", "Motor"=T6."z-Focus") -> ("Resolution-Factor"=w183:i32, "command"=w184:T4)  [unwired: 6 in, 2 out]
  n34 = Subtract(x=w51, y=w50) -> (x-y=w49:u32)
  n35 = Unbundle By Name("User") -> ("Digital-out"=w10:T8)
  n36 = call "SIAM-TMSI.vi"("Type"=enum8{"acc", "vel", "abs", "offset"}."abs", "Motor"=T6."x-Galvo") -> ("Resolution-Factor"=w122:i32, "command"=w123:T4)  [unwired: 6 in, 2 out]
  n37 = Unbundle By Name("User") -> ("Digital-out"=w58:T8)
  n38 = Subtract(x=w49, y=w48) -> (x-y=w47:u32)
  n39 = Divide(x=w169, y=w170) -> (x/y=w171:dbl)
  n40 = Multiply(x=w183, y=w171) -> (x*y=w182:dbl)
  n41 = Boolean To (0,1)(Boolean=FALSE) -> (0, 1=w12:i16)
  n42 = call "SIAM-TMSI.vi"("Type"=enum8{"acc", "vel", "abs", "offset"}."acc", "Motor"=T6."x-Galvo") -> ("Resolution-Factor"=w39:i32, "command"=w20:T4)  [unwired: 6 in, 2 out]
  n43 = Multiply(x=w21, y=w102) -> (x*y=w103:u32)
  n44 = call "SIAM-TMSI.vi"("Type"=enum8{"acc", "vel", "abs", "offset"}."acc", "Motor"=T6."Ch1") -> ("Resolution-Factor"=w32:i32, "command"=w19:T4)  [unwired: 6 in, 2 out]
  n45 = call "SIAM-TMSI.vi"("Type"=enum8{"acc", "vel", "abs", "offset"}."vel", "Motor"=T6."x-Galvo") -> ("Resolution-Factor"=w112:i32, "command"=w107:T4)  [unwired: 6 in, 2 out]
  n46 = Boolean To (0,1)(Boolean=TRUE) -> (0, 1=w60:i16)
  n47 = call "SIAM-TMSI.vi"("Type"=enum8{"acc", "vel", "abs", "offset"}."offset", "Motor"=T6."x-Galvo") -> ("Resolution-Factor"=w79:i32)  [unwired: 6 in, 3 out]
  n48 = To Unsigned Long Integer(number=w12) -> (unsigned 32bit integer=w11:u32)
  n49 = call "SIAM-TMSI.vi"("Type"=enum8{"acc", "vel", "abs", "offset"}."abs", "Motor"=T6."Ch1") -> ("Resolution-Factor"=w117:i32, "command"=w118:T4)  [unwired: 6 in, 2 out]
  n50 = To Unsigned Long Integer(number=w60) -> (unsigned 32bit integer=w59:u32)
  n51 = Divide(x=w95, y=2) -> (x/y=w94:dbl)
  n52 = Bundle By Name(cluster=w6, "Delay 10µs"=u32 0, "command"=w88, "P1"=w87) -> ()  [unwired: 1 out]
  n53 = Bundle By Name(cluster=w6, "Delay 10µs"=u32 50, "command"=w184, "P0"=w182) -> (w152:T7)
  n54 = Multiply(x=w112, y=w36) -> (x*y=w113:dbl)
  n55 = Multiply(x=w39, y=w35) -> (x*y=w27:dbl)
  n56 = Multiply(x=w122, y=w76) -> (x*y=w121:dbl)
  n57 = Logical Shift(y=w10, x=u32 1) -> (x << y=w9:u32)
  n58 = Logical Shift(y=w10, x=w11) -> (x << y=w8:u32)
  n59 = Multiply(x=w32, y=w31) -> (x*y=w25:dbl)
  n60 = Multiply(x=w79, y=w36) -> (x*y=w78:dbl)
  n61 = Logical Shift(y=w58, x=u32 1) -> (x << y=w57:u32)
  n62 = Multiply(x=w117, y=w94) -> (x*y=w116:dbl)
  n63 = Logical Shift(y=w58, x=w59) -> (x << y=w56:u32)
  n64 = Negate(x=w25) -> (-x=w26:dbl)
  n65 = Negate(x=w27) -> (-x=w28:dbl)
  n66 = Bundle By Name(cluster=w6, "Delay 10µs"=w103, "command"=w107, "P2"=w113) -> (w63:T7)
  n67 = Bundle By Name(cluster=w6, "Delay 10µs"=u32 0, "command"=w128, "P0"=w126, "P1"=w84) -> (w5:T7)
  n68 = Bundle By Name(cluster=w6, "Delay 10µs"=w47, "command"=w53, "P1"=w52) -> (w43:T7)
  n69 = Bundle By Name(cluster=w6, "Delay 10µs"=u32 0, "command"=w118, "P1"=w116) -> (w83:T7)
  n70 = Bundle By Name(cluster=w6, "command"=w20, "P3"=w27) -> (w38:T7)
  n71 = Bundle By Name(cluster=w6, "Delay 10µs"=u32 0, "command"=w123, "P1"=w121) -> (w64:T7)
  n72 = Bundle By Name(cluster=w6, "Delay 10µs"=u32 50, "command"=w162, "P0"=w160, "P1"=w146) -> (w153:T7)
  n73 = Bundle By Name(cluster=w6, "Delay 10µs"=u32 0, "command"=w92, "P1"=w91) -> (w82:T7)
  n74 = Bundle By Name(cluster=w6, "Delay 10µs"=u32 70, "command"=w101, "P0"=w96, "P1"=w100, "P2"=w97, "P5-ticket"=514) -> (w1:T7)
  n75 = Bundle By Name(cluster=w6, "command"=w19, "P3"=w25) -> (w29:T7)
  n76 = Bundle By Name(cluster=w6, "Delay 10µs"=w3, "command"=w14, "P0"=w9, "P1"=w8) -> (w2:T7)
  n77 = Bundle By Name(cluster=w6, "Delay 10µs"=w21, "command"=w20, "P3"=w28) -> (w24:T7)
  n78 = Bundle By Name(cluster=w6, "Delay 10µs"=w21, "command"=w20, "P3"=w18) -> (w17:T7)
  n79 = Bundle By Name(cluster=w6, "command"=w19, "P3"=w26) -> (w23:T7)
  n80 = Bundle By Name(cluster=w6, "Delay 10µs"=w54, "command"=w62, "P0"=w57, "P1"=w56) -> (w46:T7)
  n81 = Bundle By Name(cluster=w6, "command"=w111, "P0"=1, "P1"=1) -> (w45:T7)
  n82 = call "SIAM-ModuloPhase.vi"("GalvoFullCycle [I32]"=w78, "Predictiontick"=w50) -> ("SIAMScript"=w42:T5)  [unwired: 4 in, 1 out]
  n83 = Bundle By Name(cluster=w6, "command"=w19, "P3"=w18) -> (w16:T7)
  n84 = Bundle By Name(cluster=w45, "Delay 10µs"=w48, "P1"=0) -> (w44:T7)
  n85 = call "SIAM-TMSI.vi"("Type"=enum8{"acc", "vel", "abs", "offset"}."offset", "Motor"=T6."z-Focus") -> ("Resolution-Factor"=w177:i32, "command"=w178:T4)  [unwired: 6 in, 2 out]
  n86 = Multiply(x=w84, y=w158) -> (x*y=w150:i32)
  n87 = Multiply(x=w171, y=w146) -> (x*y=w174:dbl)
  n88 = call "SIAM-TMSI.vi"("Type"=enum8{"acc", "vel", "abs", "offset"}."abs", "Motor"=T6."x-Galvo") -> ("Resolution-Factor"=w194:i32, "command"=w193:T4)  [unwired: 6 in, 2 out]
  n89 = Negate(x=w174) -> (-x=w173:dbl)
  n90 = Decrement "z-step"(x=w150) -> (x-1=w147:i32)
  n91 = Multiply(x=w177, y=w173) -> (x*y=w176:dbl)
  n92 = Multiply(x=w194, y=w168) -> (x*y=w195:dbl)
  n93 = Bundle By Name(cluster=w6, "Delay 10µs"=u32 50, "command"=w178, "P0"=w176) -> (w172:T7)
  n94 = Bundle By Name(cluster=w6, "Delay 10µs"=u32 0, "command"=w159, "P0"=w147, "P1"=w157, "P2"=w154, "P5-ticket"=515) -> (w151:T7)
  n95 = Bundle By Name(cluster=w6, "Delay 10µs"=u32 50, "command"=w193, "P1"=w195) -> (w191:T7)
  n96 = Bundle By Name(cluster=w6, "Delay 10µs"=u32 10, "command"=w190, "P5-ticket"=112) -> (w188:T7)
  n97 = Build Array (concatenate)(w83, w64, w82, w42, w63) -> (w149:T5)
  n98 = Build Array (concatenate)(w5, w46, w45, w44, w43, w42, w38, w29, w24, w23, w17, w16, w2, w1) -> (w22:T5)
  n99 = Build Array (concatenate)(w153, w149, w22, w152, w151, w172, w191, w188) -> (w137:T5)
  "SIAMScript" <- w137
  n100 = Array Size(array=w137) -> (size(s)=→"size(s)":i32)
  "error out" <- "error in (no error)"
